vi "2.0.0_BEMF_Calibration.vi"(7 "Data in":T2, 8 "error in (no error)":errorcluster, 9 "AllControls In":T1, 10 "?":T3, 11 "Message Queue out":T4) -> (0 "error out":errorcluster, 1 "Flow":string, 2 "Data":T3, 3 "Message Queue Out":T4, 5 "Data out":T2)   [LabVIEW 2017]
uses:
  DIPC 692 Daemon API/typdef/calibration.ctl
  Depends/AMC/subVIs/TypeDefs/amc_Message Queue.ctl
  Depends/AMC/subVIs/TypeDefs/amc_Message.ctl
  Depends/Tools/Keyed Array/Tools_KeyedArray KeyedArray.ctl
  Ctrls/Data.ctl
  Ctrls/CSV_Data.ctl
  Ctrls/AllControls.ctl
panel:
  in  "Image path":path caption="路径"
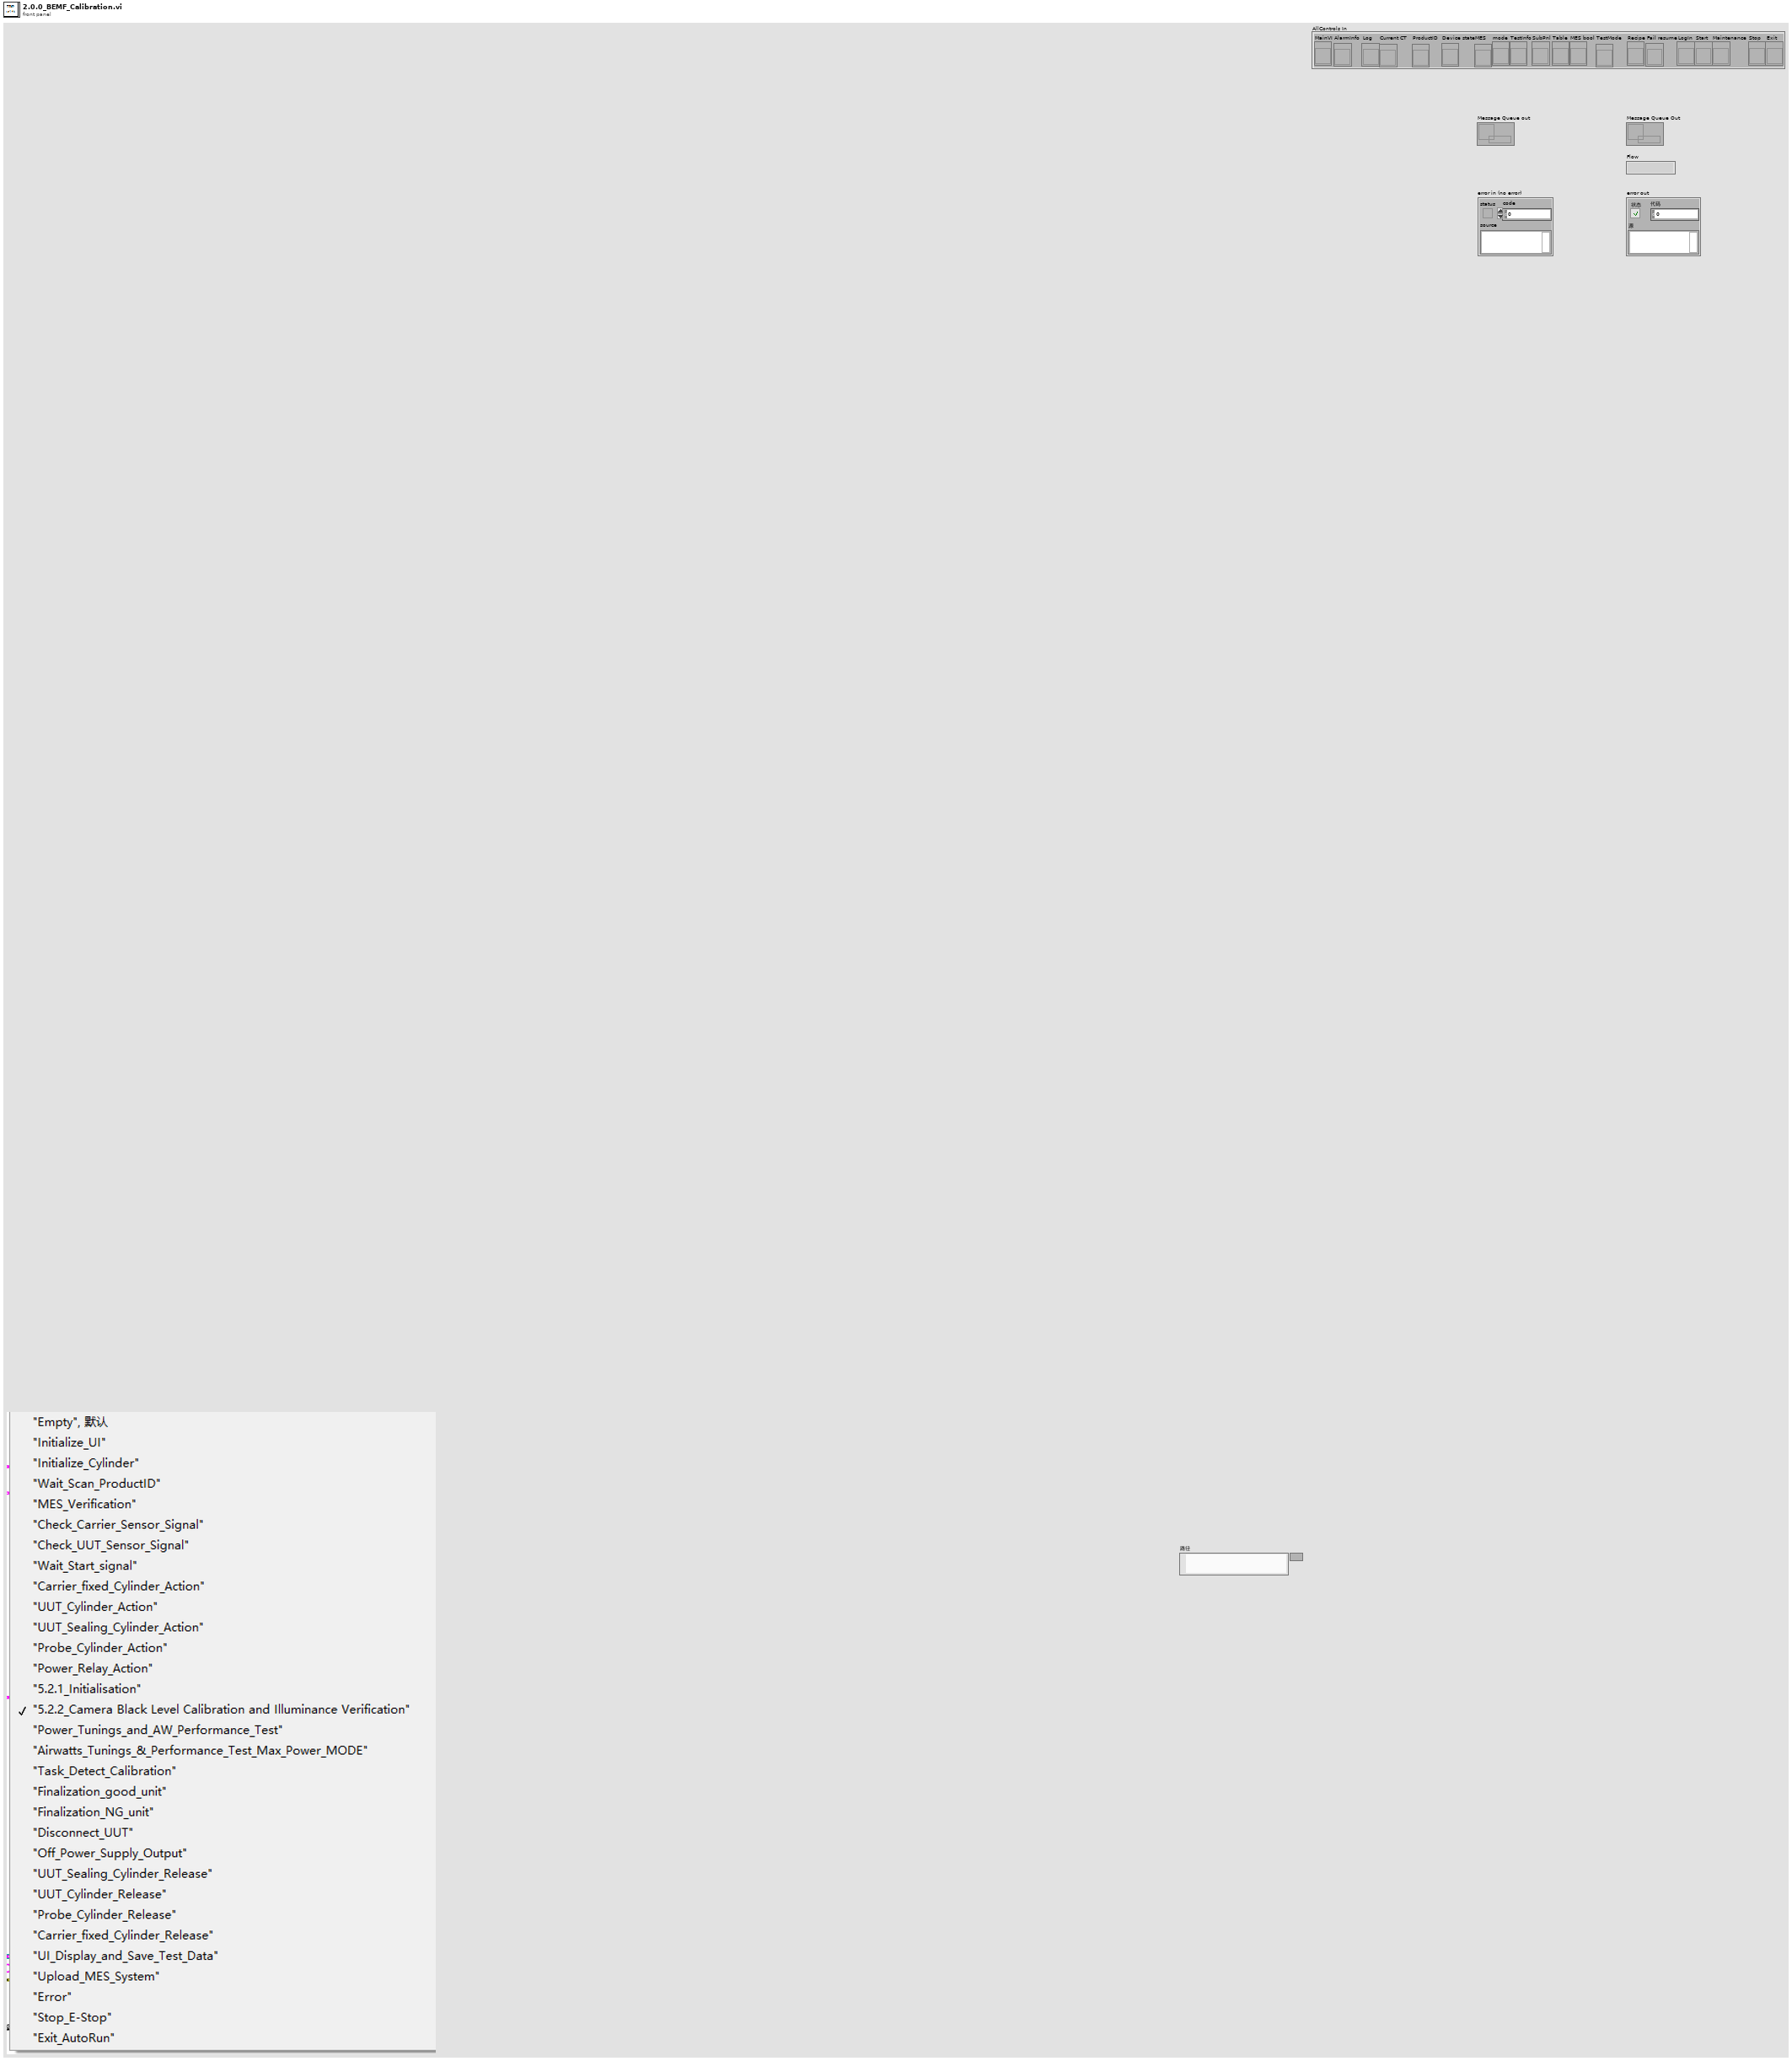
[diagram p1: front panel]
types:
  T1 = typedef "AllControls.ctl" = cluster{"MainVI":refnum<vi>, "AlarmInfo":refnum<vi>, "Log":refnum<vi>, "Current CT":refnum<vi>, "ProductID":refnum<vi>, "Device state":refnum<vi>, "MES":refnum<vi>, "mode":refnum<vi>, "TestInfo":refnum<vi>, "SubPnl":refnum<vi>, "Table":refnum<vi>, "MES bool":refnum<vi>, "TestMode":refnum<vi>, "Recipe":refnum<vi>, "Fail resume":refnum<vi>, "LogIn":refnum<vi>, "Start":refnum<vi>, "Maintenance":refnum<vi>, "Stop":refnum<vi>, "Exit":refnum<vi>}
  T2 = typedef "CSV_Data.ctl" = cluster{"Initialisation":cluster{"LMT - Connect UUT (con COM)":string, "LMT - Software Version (rrel)":string, "LMT - Write SKU file (wskuc)":string, "LMT - SKU file name":string, "Connect UUT DDM":string, "Read DDM EOL Timestamp - Mode":string, "Read DDM EOL Timestamp - Timestamp":string, "Read DDM EOL Timestamp - Rig ID":string, "Read DDM EOL Timestamp - Passmark ID":string, "Read DDM EOL Timestamp - Passmark Rev":string, "Software Version before flashing":string, "Read Hardware Serial":string, "UUT DDM SN":string, "Compare DDM SN with MES SN":string, "Backup PCBA Calibration EEPROM Response - CAL":string, "Flash Firmware Version":string, "Check SW Version":string, "Read DDM SW Version after flashing":string, "Set SKU Config":string, "Ready Status":string, "Set Device Mode to EOL":string, "DDM Parameter - Voltage":string, "DDM Parameter - Current":string, "DDM Parameter - Power":string, "DDM Parameter - Speed":string, "DDM Parameter - Pressure":string, "Tester Parameter - Voltage":string, "Tester Parameter - Current":string, "Tester Parameter - Power":string, "Tester Parameter - Ambient Pressure":string, "Tester Parameter - Ambient Temperature":string, "Calculated Parameter - DDM Pressure Corrected":string, "Calculated Parameter - DDM Real Power":string, "Calculated Parameter - Delta V":string}, "BEMF_Calibration":cluster{"Calibration Result - eol_cold_bemf_temp":string, "DDM Ambient Temp":string, "Restriction Plate Diameter":string, "Calibration Result - eol_bemf_mp_cold_coef_a":string, "Calibration Result - eol_bemf_mp_cold_coef_b":string, "Calibration Result - eol_bemf_mp_cold_coef_c":string, "Calibration Result - eol_bemf_lsi_cold_ref_coeffs":string, "Get - Calibration Result - eol_bemf_lsi_speed":string, "Get - Calibration Result - eol_bemf_lsi_integral_0":string, "Calibration Result - eol_bemf_lsi_integral_1":string, "Get - Calibration Result - eol_bemf_lsi_integral_2":string, "Get - Calibration Result - eol_cold_bemf":string, "Get - Calibration Result - eol_cold_bemf_fisf":string, "Finalise Calibration":string, "Compare -Calibration Result - eol_cold_bemf":string, "Compare -Calibration Result - eol_cold_bemf_fisf":string}, "ECO":cluster{"Reset Power Tune":string, "Reset BEMF FISF Calibration":string, "Restriction Plate Diameter":string, "ECO - Stabilisation Time":string, "ECO - DDM Parameter - Voltage":string, "ECO - DDM Parameter - Current":string, "ECO - DDM Parameter - Power":string, "ECO - DDM Parameter - Measured Power":string, "ECO - DDM Parameter - Speed":string, "ECO - DDM Parameter - Pressure":string, "ECO - Tester Parameter - Voltage":string, "ECO - Tester Parameter - Current":string, "ECO - Tester Parameter - Power":string, "ECO - Tester Parameter - Ambient Pressure":string, "ECO - Tester Parameter - Ambient Temperature":string, "ECO - Tester Parameter - Ambient Humidity":string, "ECO - Calculated Parameter - DDM Pressure Corrected":string, "ECO - Calculated Parameter - DDM Real Power":string, "ECO - Calculated Parameter - Delta V":string, "ECO - Calculated Parameter - Flowrate":string, "ECO - Calculated Parameter - Airwatt":string, "ECO - Formula":string, "PT ECO - Power Tune Mode Status":string}, "BOOST":cluster{"Restriction Plate Diameter":string, "BOOST - Stabilisation Time":string, "BOOST - DDM Parameter - Voltage":string, "BOOST - DDM Parameter - Current":string, "BOOST - DDM Parameter - Power":string, "BOOST - DDM Parameter - Measured Power":string, "BOOST - DDM Parameter - Speed":string, "BOOST - DDM Parameter - Pressure":string, "BOOST - Tester Parameter - Voltage":string, "BOOST - Tester Parameter - Current":string, "BOOST - Tester Parameter - Power":string, "BOOST - Tester Parameter - Ambient Pressure":string, "BOOST - Tester Parameter - Ambient Temperature":string, "BOOST - Tester Parameter - Ambient Humidity":string, "BOOST - Calculated Parameter - DDM Pressure Corrected":string, "BOOST - Calculated Parameter - DDM Real Power":string, "BOOST - Calculated Parameter - Delta V":string, "BOOST - Calculated Parameter - Flowrate":string, "BOOST - Calculated Parameter - Airwatt":string, "BOOST - Get AM Presence":string, "Air Muscle Turn Off Status":string, "BOOST - Air Muscle Calculated Parameter - Airwatt B":string, "BOOST - Air Muscle Calculate Airwatt Delta":string, "PT BOOST - Power Tune Mode Status":string, "Finalise Calibration":string, "ECO - Get AW Calibration value":string, "BOOST - Get AW Calibration value":string}, "MAX":cluster{"Restriction Plate Diameter":string, "MAX - Stabilisation Time":string, "Get Average Delta Tmag (LSIdelta_FISFdelta_LSItmag_FISFtmag_IIRtmag)":string, "Get Average Delta Tmag FISF":string, "MAX - DDM Parameter - Voltage":string, "MAX - DDM Parameter - Current":string, "MAX - DDM Parameter - Power":string, "MAX - DDM Parameter - Measured Power":string, "MAX - DDM Parameter - Speed":string, "MAX - DDM Parameter - Pressure":string, "MAX - Tester Parameter - Voltage":string, "MAX - Tester Parameter - Current":string, "MAX - Tester Parameter - Power":string, "MAX - Tester Parameter - Ambient Pressure":string, "MAX - Tester Parameter - Ambient Temperature":string, "MAX - Tester Parameter - Ambient Humidity":string, "MAX - Calculated Parameter - DDM Pressure Corrected":string, "MAX - Calculated Parameter - DDM Real Power":string, "MAX - Calculated Parameter - Delta V":string, "MAX - Calculated Parameter - Flowrate":string, "MAX - Calculated Parameter - Airwatt":string, "MAX_FISF_Check_Average_Delta_Tmag":string, "MAX - FISF - BEMF Finetune Result":string, "MAX tune - Delta P1":string, "MAX tune - Calculated Parameter - Airwatt":string, "Calculate Delta Airwatts - MAX finetune - Delta P2":string, "MAX finetune - DDM Parameter - Voltage":string, "MAX finetune - DDM Parameter - Current":string, "MAX finetune - DDM Parameter - Power":string, "MAX finetune - DDM Parameter - Measured Power":string, "MAX finetune - DDM Parameter - Speed":string, "MAX finetune - DDM Parameter - Pressure":string, "MAX finetune - Tester Parameter - Voltage":string, "MAX finetune - Tester Parameter - Current":string, "MAX finetune - Tester Parameter - Power":string, "MAX finetune - Tester Parameter - Ambient Pressure":string, "MAX finetune - Tester Parameter - Ambient Temperature":string, "MAX finetune - Tester Parameter - Ambient Humidity":string, "MAX finetune - Calculated Parameter - DDM Pressure Corrected":string, "MAX finetune - Calculated Parameter - DDM Real Power":string, "MAX finetune - Calculated Parameter - Delta V":string, "MAX finetune - Calculated Parameter - Flowrate":string, "MAX finetune - Calculated Parameter - Airwatt":string, "Check Derate Result":string, "Delta Tmag FISF":string, "Get Hot BEMF Result":string, "Calculate delta Pressure":string, "Finalise Calibration":string, "Calculate & Check Delta BEMF":string, "Delta P Airwatts Value":string}, "LL":cluster{"DDM Ambient Temp":string, "Restriction Plate Diameter":string, "LL - DDM Parameter - Voltage":string, "LL - DDM Parameter - Current":string, "LL - DDM Parameter - Power":string, "LL - DDM Parameter - Measured Power":string, "LL - DDM Parameter - Speed":string, "LL - DDM Parameter - Pressure":string, "LL - Tester Parameter - Voltage":string, "LL - Tester Parameter - Current":string, "LL - Tester Parameter - Power":string, "LL - DDM Real Power":string, "LL - Calibrate Task Detect LL":string}, "HL":cluster{"HL - DDM Parameter - Voltage":string, "HL - DDM Parameter - Current":string, "HL - DDM Parameter - Power":string, "HL - DDM Parameter - Measured Power":string, "HL - DDM Parameter - Speed":string, "HL - DDM Parameter - Pressure":string, "HL - Tester Parameter - Voltage":string, "HL - Tester Parameter - Current":string, "HL - Tester Parameter - Power":string, "HL - DDM Real Power":string, "HL - Calibrate Task Detect HL":string}, "LH":cluster{"Restriction Plate Diameter":string, "LH - DDM Parameter - Voltage":string, "LH - DDM Parameter - Current":string, "LH - DDM Parameter - Power":string, "LH - DDM Parameter - Measured Power":string, "LH - DDM Parameter - Speed":string, "LH - DDM Parameter - Pressure":string, "LH - Tester Parameter - Voltage":string, "LH - Tester Parameter - Current":string, "LH - Tester Parameter - Power":string, "LH - DDM Real Power":string, "LH - Calibrate Task Detect LH":string}, "HH":cluster{"HH - DDM Parameter - Voltage":string, "HH - DDM Parameter - Current":string, "HH - DDM Parameter - Power":string, "HH - DDM Parameter - Measured Power":string, "HH - DDM Parameter - Speed":string, "HH - DDM Parameter - Pressure":string, "HH - Tester Parameter - Voltage":string, "HH - Tester Parameter - Current":string, "HH - Tester Parameter - Power":string, "HH - DDM Real Power":string, "HH - Calibrate Task Detect HH":string}, "Inlet Blockage Calibration":cluster{"Inlet Blockage Calibration - DDM Parameter - Voltage":string, "Inlet Blockage Calibration - DDM Parameter - Current":string, "Inlet Blockage Calibration - DDM Parameter - Power":string, "Inlet Blockage Calibration - DDM Parameter - Measured Power":string, "Inlet Blockage Calibration - DDM Parameter - Speed":string, "Inlet Blockage Calibration - DDM Parameter - Pressure":string, "Inlet Blockage Calibration - Tester Parameter - Voltage":string, "Inlet Blockage Calibration - Tester Parameter - Current":string, "Inlet Blockage Calibration - Tester Parameter - Power":string, "Inlet Blockage Calibration - DDM Real Power":string, "Calibration Inlet Blockage_E":string, "Finalise Calibration":string, "Get Task Detect LL":string, "Get Task Detect HL":string, "Get Task Detect LH":string, "Get Task Detect HH":string, "Calibration Inlet Blockage":string, "Calibration eol cold bemf temp":string}, "GOOD":cluster{"GOOD UNIT - Clear EEPROM Error Log":string, "GOOD UNIT - Write Product Timestamp - Mode":string, "GOOD UNIT - Write Product Timestamp - Timestamp":string, "GOOD UNIT - Write Product Timestamp - Rig ID":string, "GOOD UNIT - Write Product Timestamp - Passmark ID":string, "GOOD UNIT - Write Product Timestamp - Passmark Rev":string, "GOOD UNIT - Set Device Mode to PROD":string, "GOOD UNIT - Backup PCBA Calibration EEPROM Response":string, "GOOD UNIT - Check Security Bit":string, "GOOD UNIT - Set Calibration Lock":string, "GOOD UNIT - Get_Calibration_Lock":string, "GOOD UNIT - Disconnect UUT":string}, "NG":cluster{"NG UNIT - Read NVM Error":string, "NG UNIT - Set Device Mode to FCT":string, "NG UNIT - Backup PCBA Calibration EEPROM Response - CAL":string, "NG UNIT - Backup PCBA Calibration EEPROM Response - ERROR":string, "NG UNIT - Backup PCBA Calibration EEPROM Response - USAGE":string, "NG UNIT - Disconnect UUT":string}, "SN":string, "Table":string[][], "Count":cluster{"Total":i32, "OK":i32, "NG":i32, "Yield":dbl}, "Start Time":timestamp, "daemon reference":refnum<k5>, "CT":dbl, "Config":string[][], "OK/NG":bool, "Station ID":string, "MES DDM SN":string, "MES PCBA SN":string, "Retest":string, "Lux":string, "Initialisation_Status":cluster{"LMT - Connect UUT (con COM)":string, "LMT - Software Version (rrel)":string, "LMT - Write SKU file (wskuc)":string, "LMT - SKU file name":string, "Connect UUT DDM":string, "Read DDM EOL Timestamp - Mode":string, "Read DDM EOL Timestamp - Timestamp":string, "Read DDM EOL Timestamp - Rig ID":string, "Read DDM EOL Timestamp - Passmark ID":string, "Read DDM EOL Timestamp - Passmark Rev":string, "Software Version before flashing":string, "Read Hardware Serial":string, "UUT DDM SN":string, "Compare DDM SN with MES SN":string, "Backup PCBA Calibration EEPROM Response - CAL":string, "Flash Firmware Version":string, "Check SW Version":string, "Read DDM SW Version after flashing":string, "Set SKU Config":string, "Ready Status":string, "Set Device Mode to EOL":string, "DDM Parameter - Voltage":string, "DDM Parameter - Current":string, "DDM Parameter - Power":string, "DDM Parameter - Speed":string, "DDM Parameter - Pressure":string, "Tester Parameter - Voltage":string, "Tester Parameter - Current":string, "Tester Parameter - Power":string, "Tester Parameter - Ambient Pressure":string, "Tester Parameter - Ambient Temperature":string, "Calculated Parameter - DDM Pressure Corrected":string, "Calculated Parameter - DDM Real Power":string, "Calculated Parameter - Delta V":string}, "BEMF_Calibration_Status":cluster{"Calibration Result - eol_cold_bemf_temp":string, "DDM Ambient Temp":string, "Restriction Plate Diameter":string, "Calibration Result - eol_bemf_mp_cold_coef_a":string, "Calibration Result - eol_bemf_mp_cold_coef_b":string, "Calibration Result - eol_bemf_mp_cold_coef_c":string, "Calibration Result - eol_bemf_lsi_cold_ref_coeffs":string, "Get - Calibration Result - eol_bemf_lsi_speed":string, "Get - Calibration Result - eol_bemf_lsi_integral_0":string, "Calibration Result - eol_bemf_lsi_integral_1":string, "Get - Calibration Result - eol_bemf_lsi_integral_2":string, "Get - Calibration Result - eol_cold_bemf":string, "Get - Calibration Result - eol_cold_bemf_fisf":string, "Finalise Calibration":string, "Compare -Calibration Result - eol_cold_bemf":string, "Compare -Calibration Result - eol_cold_bemf_fisf":string}, "ECO_Status":cluster{"Reset Power Tune":string, "Reset BEMF FISF Calibration":string, "Restriction Plate Diameter":string, "ECO - Stabilisation Time":string, "ECO - DDM Parameter - Voltage":string, "ECO - DDM Parameter - Current":string, "ECO - DDM Parameter - Power":string, "ECO - DDM Parameter - Measured Power":string, "ECO - DDM Parameter - Speed":string, "ECO - DDM Parameter - Pressure":string, "ECO - Tester Parameter - Voltage":string, "ECO - Tester Parameter - Current":string, "ECO - Tester Parameter - Power":string, "ECO - Tester Parameter - Ambient Pressure":string, "ECO - Tester Parameter - Ambient Temperature":string, "ECO - Tester Parameter - Ambient Humidity":string, "ECO - Calculated Parameter - DDM Pressure Corrected":string, "ECO - Calculated Parameter - DDM Real Power":string, "ECO - Calculated Parameter - Delta V":string, "ECO - Calculated Parameter - Flowrate":string, "ECO - Calculated Parameter - Airwatt":string, "ECO - Formula":string, "PT ECO - Power Tune Mode Status":string}, "BOOST_Status":cluster{"Restriction Plate Diameter":string, "BOOST - Stabilisation Time":string, "BOOST - DDM Parameter - Voltage":string, "BOOST - DDM Parameter - Current":string, "BOOST - DDM Parameter - Power":string, "BOOST - DDM Parameter - Measured Power":string, "BOOST - DDM Parameter - Speed":string, "BOOST - DDM Parameter - Pressure":string, "BOOST - Tester Parameter - Voltage":string, "BOOST - Tester Parameter - Current":string, "BOOST - Tester Parameter - Power":string, "BOOST - Tester Parameter - Ambient Pressure":string, "BOOST - Tester Parameter - Ambient Temperature":string, "BOOST - Tester Parameter - Ambient Humidity":string, "BOOST - Calculated Parameter - DDM Pressure Corrected":string, "BOOST - Calculated Parameter - DDM Real Power":string, "BOOST - Calculated Parameter - Delta V":string, "BOOST - Calculated Parameter - Flowrate":string, "BOOST - Calculated Parameter - Airwatt":string, "BOOST - Get AM Presence":string, "Air Muscle Turn Off Status":string, "BOOST - Air Muscle Calculated Parameter - Airwatt B":string, "BOOST - Air Muscle Calculate Airwatt Delta":string, "PT BOOST - Power Tune Mode Status":string, "Finalise Calibration":string, "ECO - Get AW Calibration value":string, "BOOST - Get AW Calibration value":string}, "MAX_Status":cluster{"Restriction Plate Diameter":string, "MAX - Stabilisation Time":string, "Get Average Delta Tmag (LSIdelta_FISFdelta_LSItmag_FISFtmag_IIRtmag)":string, "Get Average Delta Tmag FISF":string, "MAX - DDM Parameter - Voltage":string, "MAX - DDM Parameter - Current":string, "MAX - DDM Parameter - Power":string, "MAX - DDM Parameter - Measured Power":string, "MAX - DDM Parameter - Speed":string, "MAX - DDM Parameter - Pressure":string, "MAX - Tester Parameter - Voltage":string, "MAX - Tester Parameter - Current":string, "MAX - Tester Parameter - Power":string, "MAX - Tester Parameter - Ambient Pressure":string, "MAX - Tester Parameter - Ambient Temperature":string, "MAX - Tester Parameter - Ambient Humidity":string, "MAX - Calculated Parameter - DDM Pressure Corrected":string, "MAX - Calculated Parameter - DDM Real Power":string, "MAX - Calculated Parameter - Delta V":string, "MAX - Calculated Parameter - Flowrate":string, "MAX - Calculated Parameter - Airwatt":string, "MAX_FISF_Check_Average_Delta_Tmag":string, "MAX - FISF - BEMF Finetune Result":string, "MAX tune - Delta P1":string, "MAX tune - Calculated Parameter - Airwatt":string, "Calculate Delta Airwatts - MAX finetune - Delta P2":string, "MAX finetune - DDM Parameter - Voltage":string, "MAX finetune - DDM Parameter - Current":string, "MAX finetune - DDM Parameter - Power":string, "MAX finetune - DDM Parameter - Measured Power":string, "MAX finetune - DDM Parameter - Speed":string, "MAX finetune - DDM Parameter - Pressure":string, "MAX finetune - Tester Parameter - Voltage":string, "MAX finetune - Tester Parameter - Current":string, "MAX finetune - Tester Parameter - Power":string, "MAX finetune - Tester Parameter - Ambient Pressure":string, "MAX finetune - Tester Parameter - Ambient Temperature":string, "MAX finetune - Tester Parameter - Ambient Humidity":string, "MAX finetune - Calculated Parameter - DDM Pressure Corrected":string, "MAX finetune - Calculated Parameter - DDM Real Power":string, "MAX finetune - Calculated Parameter - Delta V":string, "MAX finetune - Calculated Parameter - Flowrate":string, "MAX finetune - Calculated Parameter - Airwatt":string, "Check Derate Result":string, "Delta Tmag FISF":string, "Get Hot BEMF Result":string, "Calculate delta Pressure":string, "Finalise Calibration":string, "Calculate & Check Delta BEMF":string, "Delta P Airwatts Value":string}, "LL_Status":cluster{"DDM Ambient Temp":string, "Restriction Plate Diameter":string, "LL - DDM Parameter - Voltage":string, "LL - DDM Parameter - Current":string, "LL - DDM Parameter - Power":string, "LL - DDM Parameter - Measured Power":string, "LL - DDM Parameter - Speed":string, "LL - DDM Parameter - Pressure":string, "LL - Tester Parameter - Voltage":string, "LL - Tester Parameter - Current":string, "LL - Tester Parameter - Power":string, "LL - DDM Real Power":string, "LL - Calibrate Task Detect LL":string}, "HL_Status":cluster{"HL - DDM Parameter - Voltage":string, "HL - DDM Parameter - Current":string, "HL - DDM Parameter - Power":string, "HL - DDM Parameter - Measured Power":string, "HL - DDM Parameter - Speed":string, "HL - DDM Parameter - Pressure":string, "HL - Tester Parameter - Voltage":string, "HL - Tester Parameter - Current":string, "HL - Tester Parameter - Power":string, "HL - DDM Real Power":string, "HL - Calibrate Task Detect HL":string}, "LH_Status":cluster{"Restriction Plate Diameter":string, "LH - DDM Parameter - Voltage":string, "LH - DDM Parameter - Current":string, "LH - DDM Parameter - Power":string, "LH - DDM Parameter - Measured Power":string, "LH - DDM Parameter - Speed":string, "LH - DDM Parameter - Pressure":string, "LH - Tester Parameter - Voltage":string, "LH - Tester Parameter - Current":string, "LH - Tester Parameter - Power":string, "LH - DDM Real Power":string, "LH - Calibrate Task Detect LH":string}, "HH_Status":cluster{"HH - DDM Parameter - Voltage":string, "HH - DDM Parameter - Current":string, "HH - DDM Parameter - Power":string, "HH - DDM Parameter - Measured Power":string, "HH - DDM Parameter - Speed":string, "HH - DDM Parameter - Pressure":string, "HH - Tester Parameter - Voltage":string, "HH - Tester Parameter - Current":string, "HH - Tester Parameter - Power":string, "HH - DDM Real Power":string, "HH - Calibrate Task Detect HH":string}, "Inlet Blockage Calibration_Status":cluster{"Inlet Blockage Calibration - DDM Parameter - Voltage":string, "Inlet Blockage Calibration - DDM Parameter - Current":string, "Inlet Blockage Calibration - DDM Parameter - Power":string, "Inlet Blockage Calibration - DDM Parameter - Measured Power":string, "Inlet Blockage Calibration - DDM Parameter - Speed":string, "Inlet Blockage Calibration - DDM Parameter - Pressure":string, "Inlet Blockage Calibration - Tester Parameter - Voltage":string, "Inlet Blockage Calibration - Tester Parameter - Current":string, "Inlet Blockage Calibration - Tester Parameter - Power":string, "Inlet Blockage Calibration - DDM Real Power":string, "Calibration Inlet Blockage_E":string, "Finalise Calibration":string, "Get Task Detect LL":string, "Get Task Detect HL":string, "Get Task Detect LH":string, "Get Task Detect HH":string, "Calibration Inlet Blockage":string, "Calibration eol cold bemf temp":string}, "GOOD_Status":cluster{"GOOD UNIT - Clear EEPROM Error Log":string, "GOOD UNIT - Write Product Timestamp - Mode":string, "GOOD UNIT - Write Product Timestamp - Timestamp":string, "GOOD UNIT - Write Product Timestamp - Rig ID":string, "GOOD UNIT - Write Product Timestamp - Passmark ID":string, "GOOD UNIT - Write Product Timestamp - Passmark Rev":string, "GOOD UNIT - Set Device Mode to PROD":string, "GOOD UNIT - Backup PCBA Calibration EEPROM Response":string, "GOOD UNIT - Check Security Bit":string, "GOOD UNIT - Set Calibration Lock":string, "GOOD UNIT - Get_Calibration_Lock":string, "GOOD UNIT - Disconnect UUT":string}, "NG_Status":cluster{"NG UNIT - Read NVM Error":string, "NG UNIT - Set Device Mode to FCT":string, "NG UNIT - Backup PCBA Calibration EEPROM Response - CAL":string, "NG UNIT - Backup PCBA Calibration EEPROM Response - ERROR":string, "NG UNIT - Backup PCBA Calibration EEPROM Response - USAGE":string, "NG UNIT - Disconnect UUT":string}, "SKU":string, "Plate_Diameter":string, "Alarm":string}
  T3 = typedef "Data.ctl" = cluster{"Initialisation":cluster{"DDM_Parameter":dbl[], "DDM_Parameter_status":bool[], "Get_Tester_Parameter":dbl[], "Get_Tester_Parameter_status":bool[], "Cal_Tester_Parameter":dbl[], "Cal_Tester_Parameter_status":bool[], "sw_version_before_status":bool, "sw_version_after_status":bool, "Set_SKU_Config_With_LMT_status":bool, "FCT_timestamp_status":bool, "LMT_Connect_to_UUT_status":bool}, "BEMF_Calibration":cluster{"Read_ambient_temperature":dbl, "Calibration_Vaule":dbl[], "Calibration_Vaule _B":dbl[], "Calibration_Vaule_status":bool[], "Calibration_Vaule_B_status":bool[]}, "ECO":cluster{"DDM_Parameter":dbl[], "DDM_Parameter_status":bool[], "Get_Tester_Parameter":dbl[], "Get_Tester_Parameter_status":bool[], "Cal_Tester_Parameter":dbl[], "Cal_Tester_Parameter_status":bool[], "DDM_Parameter_after_power_tune":dbl[], "Get_Tester_Parameter_after_power_tune":dbl[], "Cal_Tester_Parameter_after_power_tune":dbl[], "Cal_Tester_Parameter_after_power_tune_status":bool[], "Delta_P":dbl}, "BOOST":cluster{"DDM_Parameter":dbl[], "DDM_Parameter_status":bool[], "Get_Tester_Parameter":dbl[], "Get_Tester_Parameter_status":bool[], "Cal_Tester_Parameter":dbl[], "Cal_Tester_Parameter_status":bool[], "DDM_Parameter_after_power_tune":dbl[], "Get_Tester_Parameter_after_power_tune":dbl[], "Cal_Tester_Parameter_after_power_tune":dbl[], "Cal_Tester_Parameter_after_power_tune_status":bool[], "airwatts_am_off":dbl, "AW_Delta_(AM_on_and_off)":dbl, "AW_Delta_(AM_on_and_off)_Status":bool, "Delta_P":dbl}, "MAX":cluster{"Average_Tmag_Data":cluster{"LSI Delta in degC":dbl, "FISF Delta in degc":dbl, "LSI Tmag in degC":dbl, "Fisf Tmag in degC":dbl, "IIR Tmag in degC":dbl}, "DDM_Parameter":dbl[], "DDM_Parameter_status":bool[], "Get_Tester_Parameter":dbl[], "Get_Tester_Parameter_status":bool[], "Cal_Tester_Parameter":dbl[], "BEMF_Finetune":cluster{"eol_bemf_mp_cold_coef_c":dbl, "eol_cold_bemf_fisf_offset":dbl}, "AW_Tune":cluster{"delta_P1":dbl, "delta_P_Setting":dbl}, "DDM_Parameter_after_Airwatts_Tune":dbl[], "Get_Tester_Parameter_after_Airwatts_Tune":dbl[], "Cal_Tester_Parameter_after_Airwatts_Tune":dbl[], "DDM_Parameter_after_Airwatts_Finetune":dbl[], "Get_Tester_Parameter_after_Airwatts_Finetune":dbl[], "Cal_Tester_Parameter_after_Airwatts_Finetune":dbl[], "AW_Finetune":cluster{"delta_P2":dbl, "delta_P_Setting":dbl}, "Delta_Tmag_after_tune":cluster{"LSI Delta in degC":dbl, "FISF Delta in degc":dbl, "LSI Tmag in degC":dbl, "Fisf Tmag in degC":dbl, "IIR Tmag in degC":dbl}, "Hot Bemf in mV":dbl, "DDM_Pressure":dbl, "Delta_Pressure":dbl, " Cold Bemf in mV":dbl, " delta Bemf":dbl, " delta p":dbl, "Delta_Pressure_status":bool, " delta Bemf_status":bool, "LSI Delta in degC_status":bool, "FISF Delta in degc_status":bool, "Max_check_derate_status_status":bool, "Average_All_data":dbl[][], "Average_Tmag_Data_status":bool[], "Average_Tmag_Data_after_tune_status":bool[], "Cal_Tester_Parameter_status":bool[], "Cal_Tester_Parameter_status_after_Airwatts_Tune":bool[], "Cal_Tester_Parameter_status_after_Airwatts_FineTune":bool[]}, "Task_Detect_Calib":cluster{"LL":cluster{"DDM_Parameter":dbl[], "DDM_Parameter_status":bool[], "Get_Tester_Parameter":dbl[], "Get_Tester_Parameter_status":bool[], "Set_task_detect_A":dbl, "Set_task_detect_A_Status":bool}, "HL":cluster{"DDM_Parameter":dbl[], "DDM_Parameter_status":bool[], "Get_Tester_Parameter":dbl[], "Get_Tester_Parameter_status":bool[], "Set_task_detect_B":dbl, "Set_task_detect_B_Status":bool}, "LH":cluster{"DDM_Parameter":dbl[], "DDM_Parameter_status":bool[], "Get_Tester_Parameter":dbl[], "Get_Tester_Parameter_status":bool[], "Set_task_detect_C":dbl, "Set_task_detect_C_Status":bool}, "HH":cluster{"DDM_Parameter":dbl[], "DDM_Parameter_status":bool[], "Get_Tester_Parameter":dbl[], "Get_Tester_Parameter_status":bool[], "Set_task_detect_D":dbl, "Read_and_check_calibration_Status":bool[], "Set_task_detect_D_Status":bool}, "Get_eol_inlet_blockage_E":dbl, "Calib_vaule":cluster{"Get_task_detect_LL":dbl, "Get_task_detect_HL":dbl, "Get_task_detect_LH":dbl, "Get_task_detect_HH":dbl, "eol_inlet_blockage":dbl, "eol_code_bemf_temp":dbl}, "calibrated temp":dbl, "Inlet_Blockage_Calibration":cluster{"DDM_Parameter":dbl[], "DDM_Parameter_status":bool[], "Get_Tester_Parameter":dbl[], "Get_Tester_Parameter_status":bool[]}, "Get_eol_inlet_blockage_E_Status":bool}, "good":cluster{"Write_Product_TS":cluster{"TIMESTAMP":i64, "RIG_ID":i64, "PASSMARK_ID":i64, "PASSMARK_REV":i64}, "Read_Product_TS":cluster{"TIMESTAMP":i64, "RIG_ID":i64, "PASSMARK_ID":i64, "PASSMARK_REV":i64}, "Good_Check_Secuity_Bit_Stauts":bool}}
  T4 = typedef "amc_Message Queue.ctl" = refnum<queue>
  T5 = typedef "HD Config.ctl" = cluster{" PC":cluster{"PC Address":u8[], "PC Port":i32}, "FCO":cluster{"COM":refnum<visa-resource-name>, "Baudrate":u32}, "DC Power ":cluster{"COM":refnum<visa-resource-name>, "Baudrate":u32}, "PW3336":cluster{"COM":refnum<visa-resource-name>, "Baudrate":u32}, "Lefoo":cluster{"COM":refnum<visa-resource-name>, "Baudrate":u32}, "Tempt&Hum":cluster{"COM":refnum<visa-resource-name>, "Baudrate":u32}, "DIPC":cluster{"COM":refnum<visa-resource-name>}, "Daemon":cluster{"IP Address":string, "Port":u16, "Retry":u16}, "Motor":cluster{"COM":refnum<visa-resource-name>, "Baudrate":u32}, "Fail_resume_mode":bool, "GRR":bool}
  T6 = cluster{"getVersion":string, "Start Test mode":string, "Start camera test mode P1":string, "get one RAW Image":string, "Start camera test mode P0":string, "Stop Test Mode":string, "Stop Camera":string}
  T7 = typedef "calibration.ctl" = string
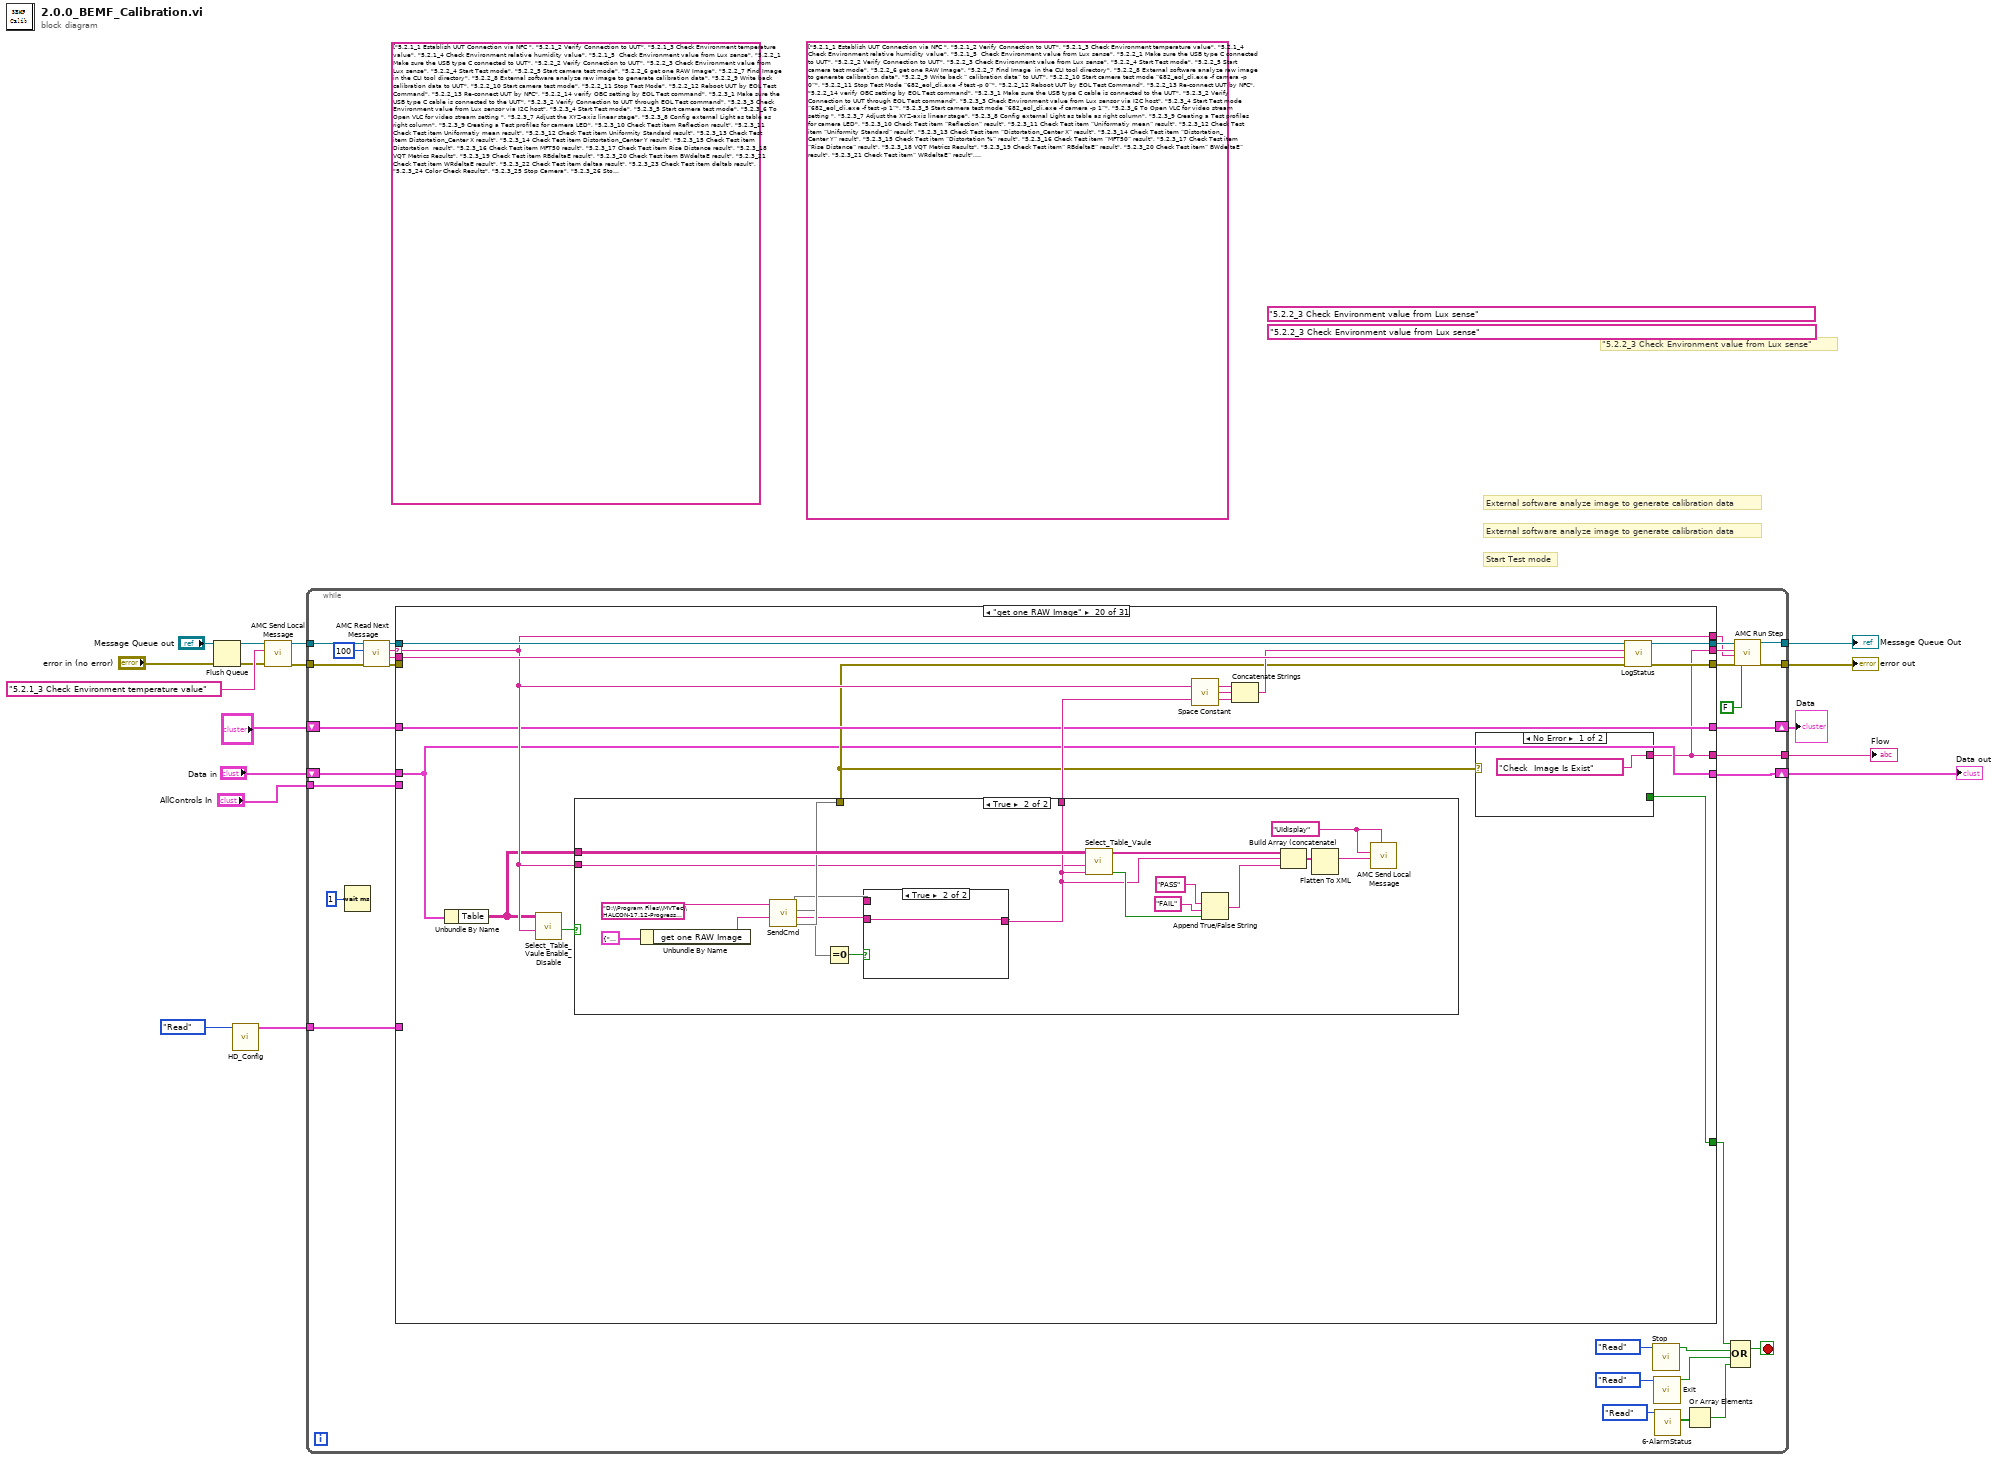
[diagram p0: block diagram]
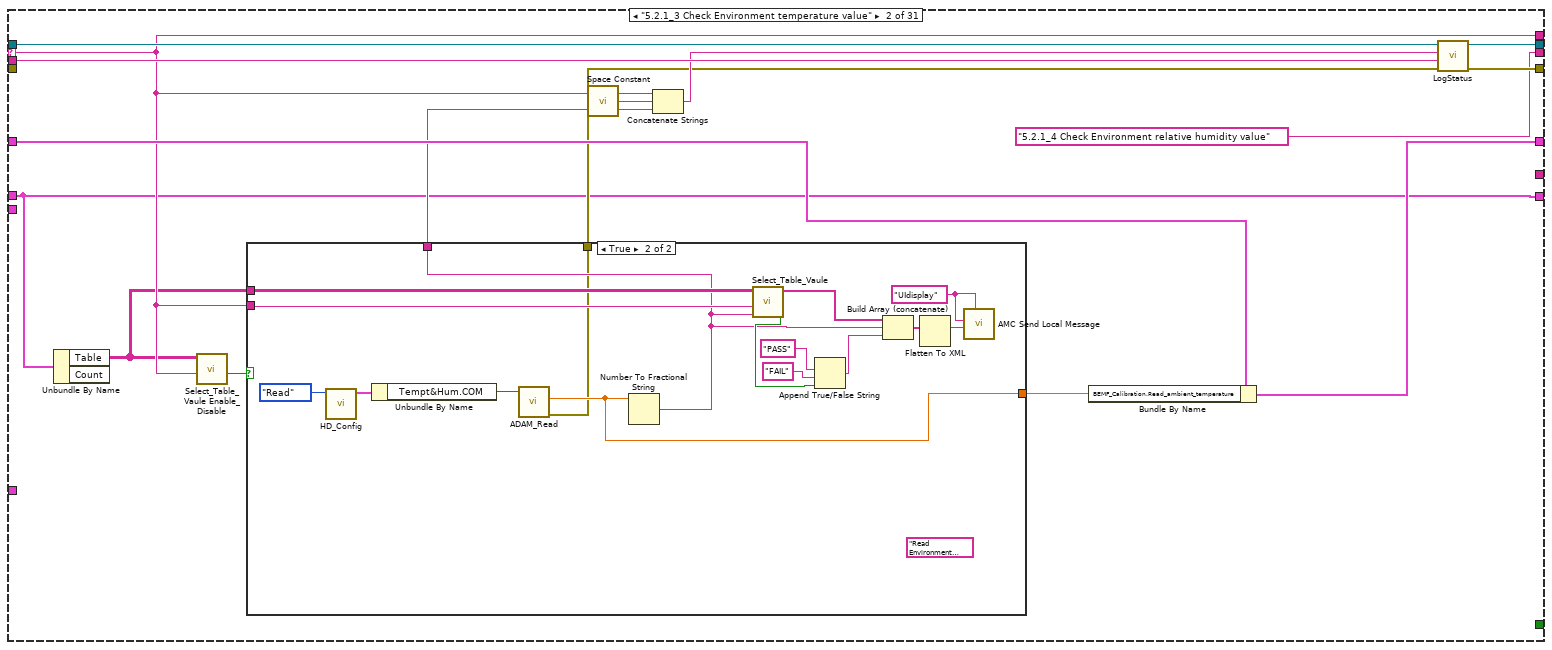
[diagram p3: hidden frame]
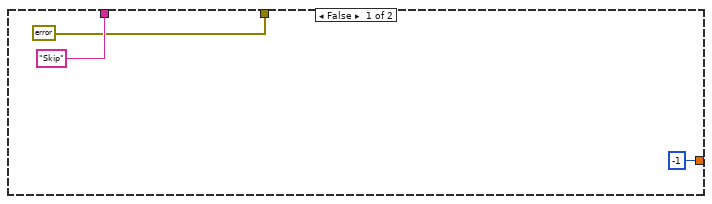
[diagram p4: hidden frame]
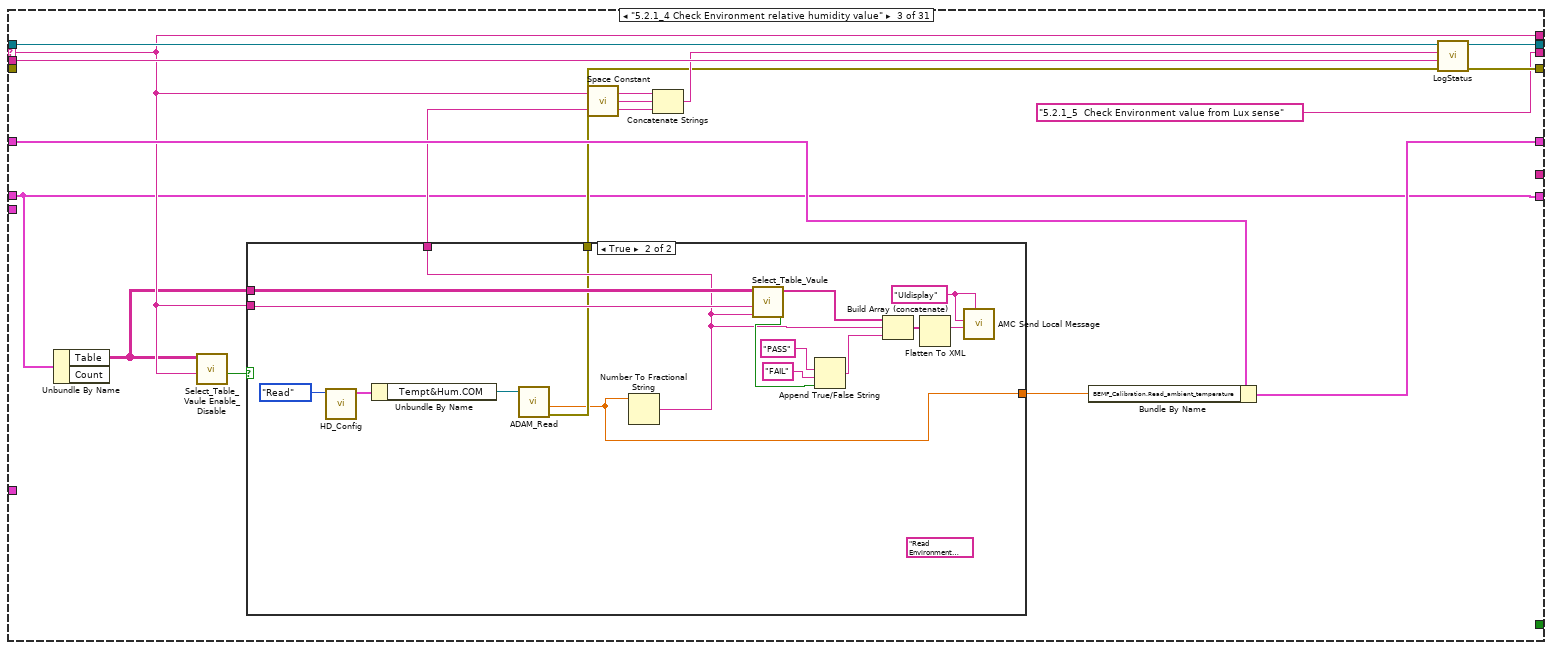
[diagram p5: hidden frame]
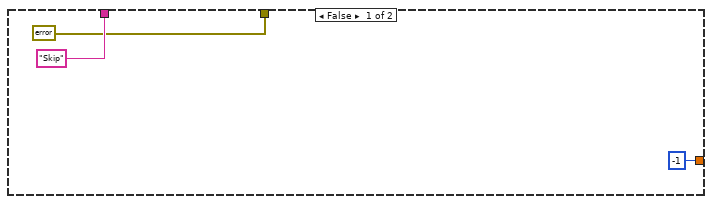
[diagram p6: hidden frame]
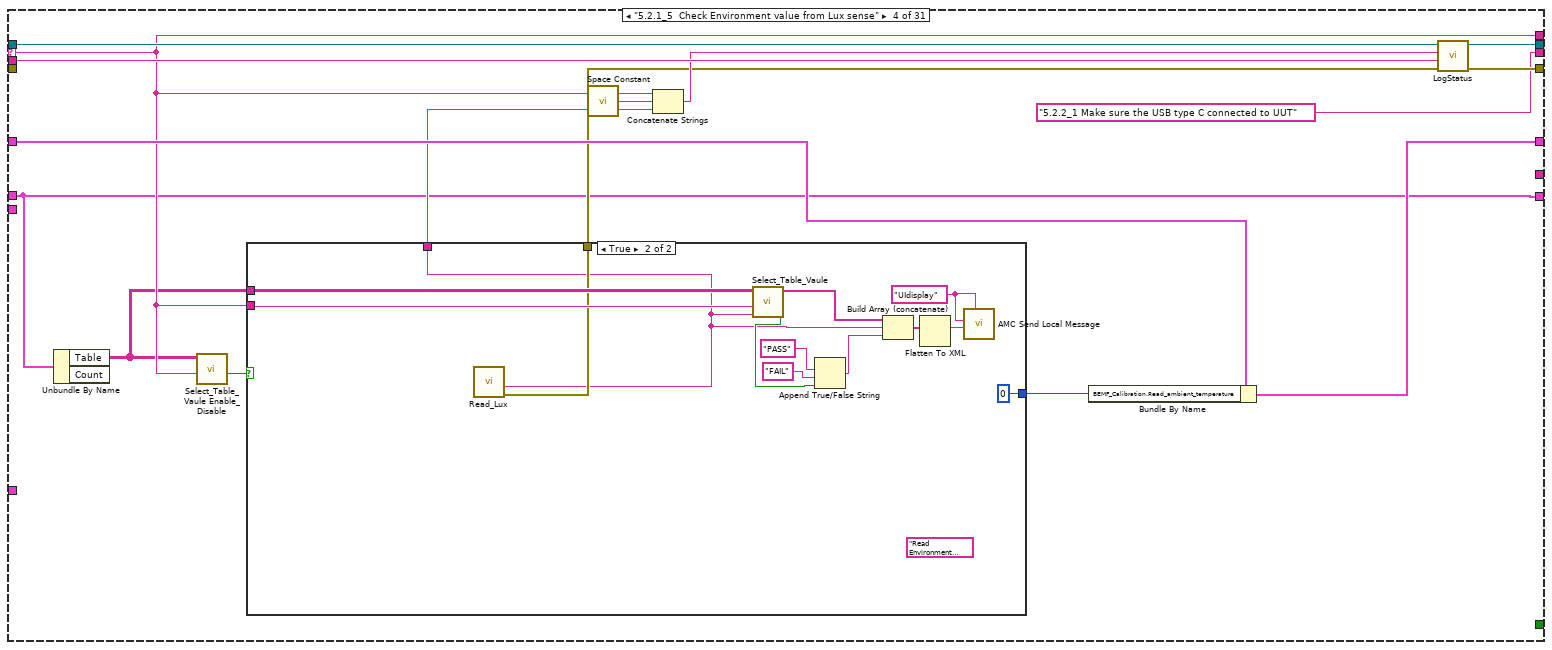
[diagram p7: hidden frame]
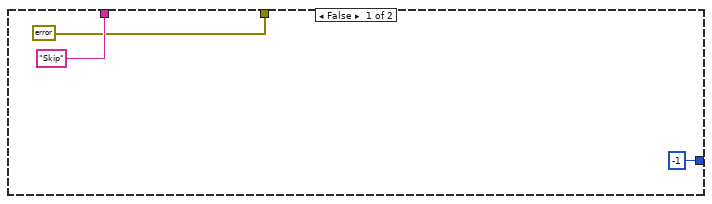
[diagram p8: hidden frame]
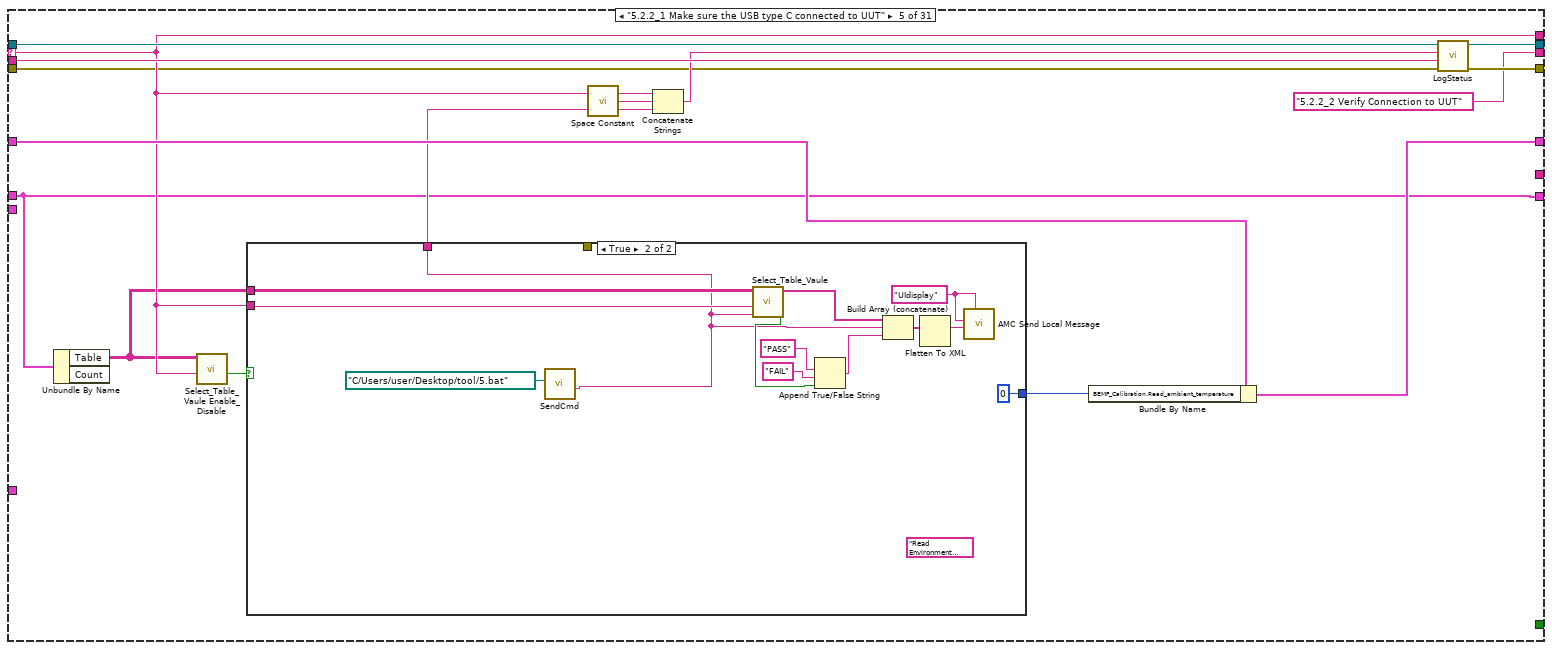
[diagram p9: hidden frame]
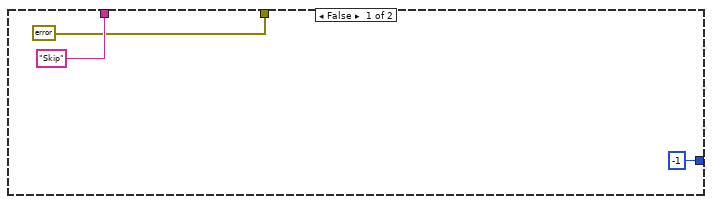
[diagram p10: hidden frame]
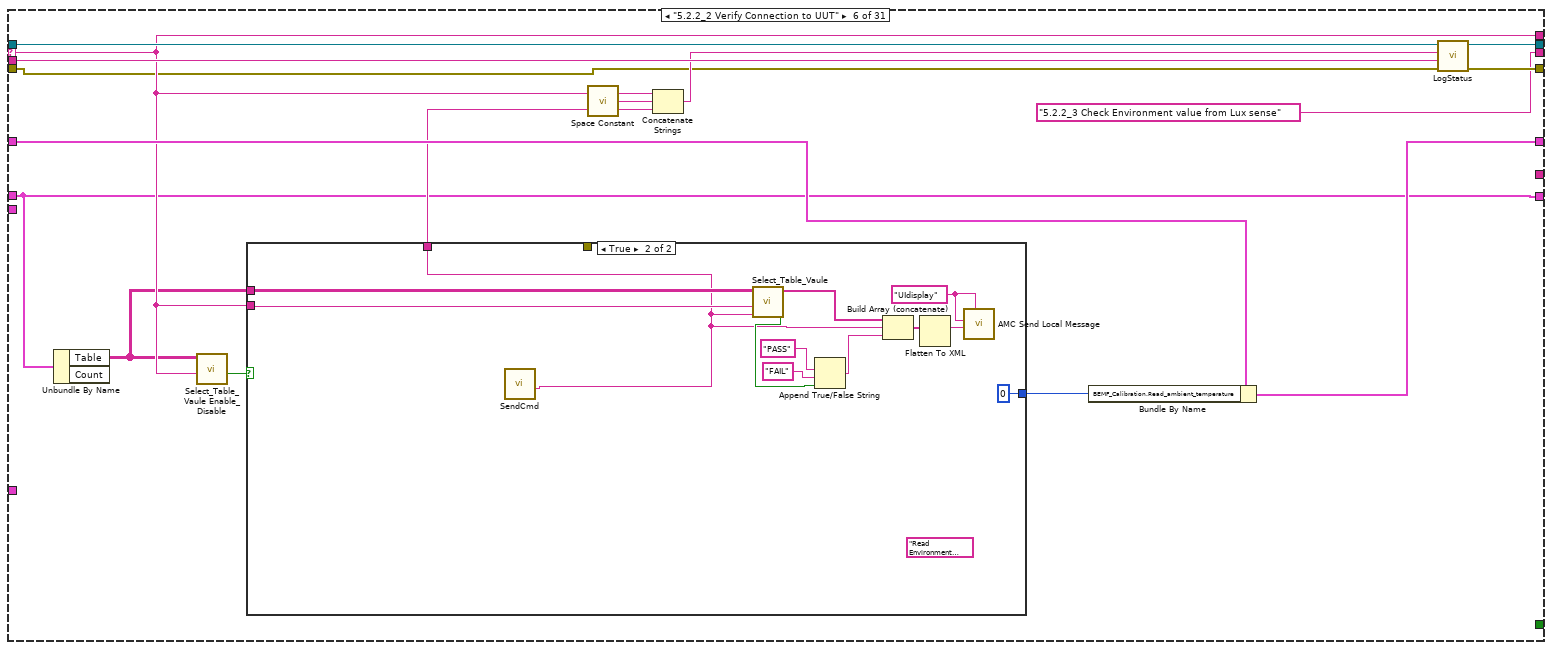
[diagram p11: hidden frame]
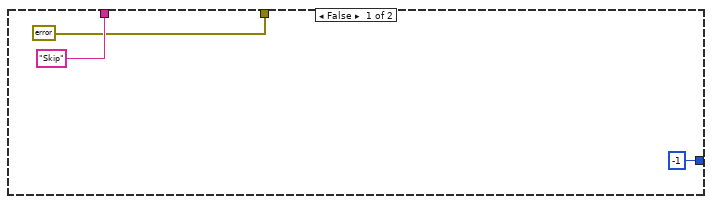
[diagram p12: hidden frame]
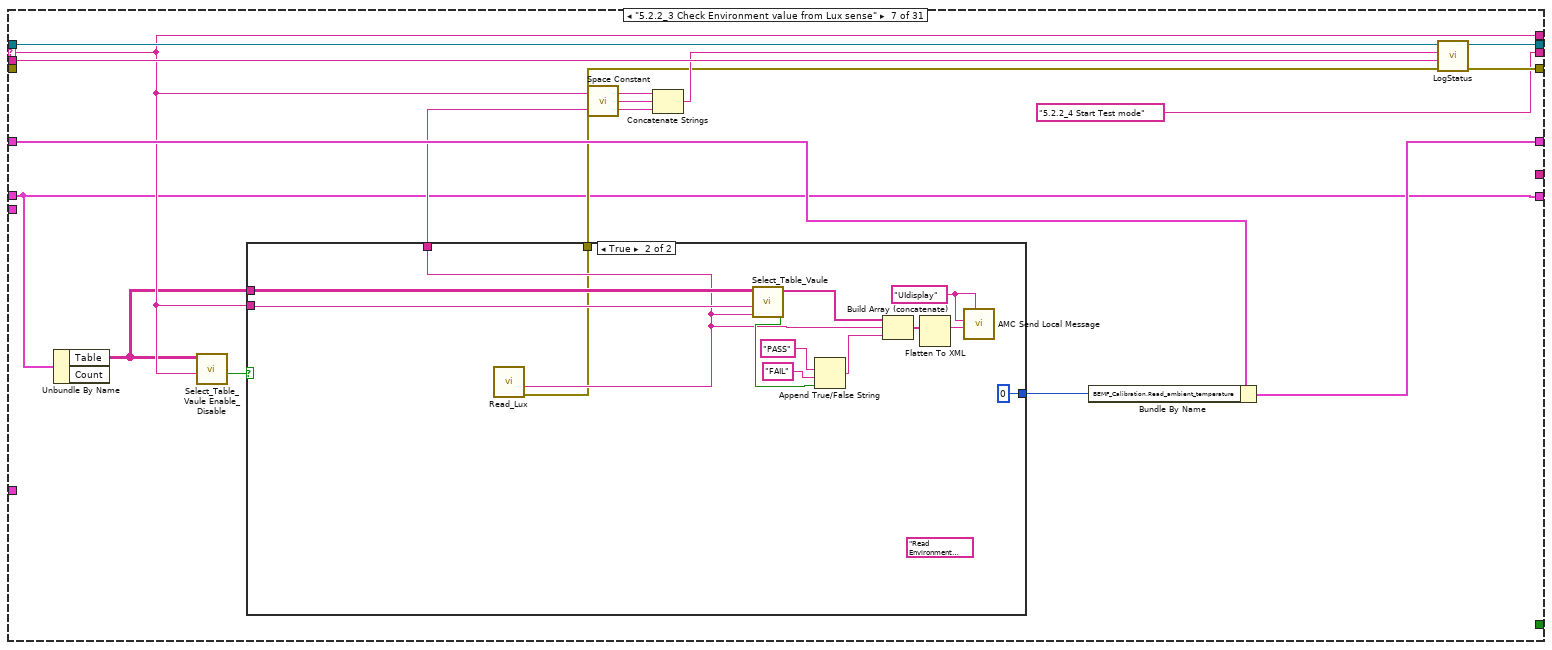
[diagram p13: hidden frame]
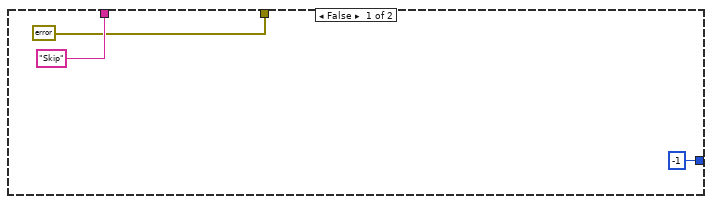
[diagram p14: hidden frame]
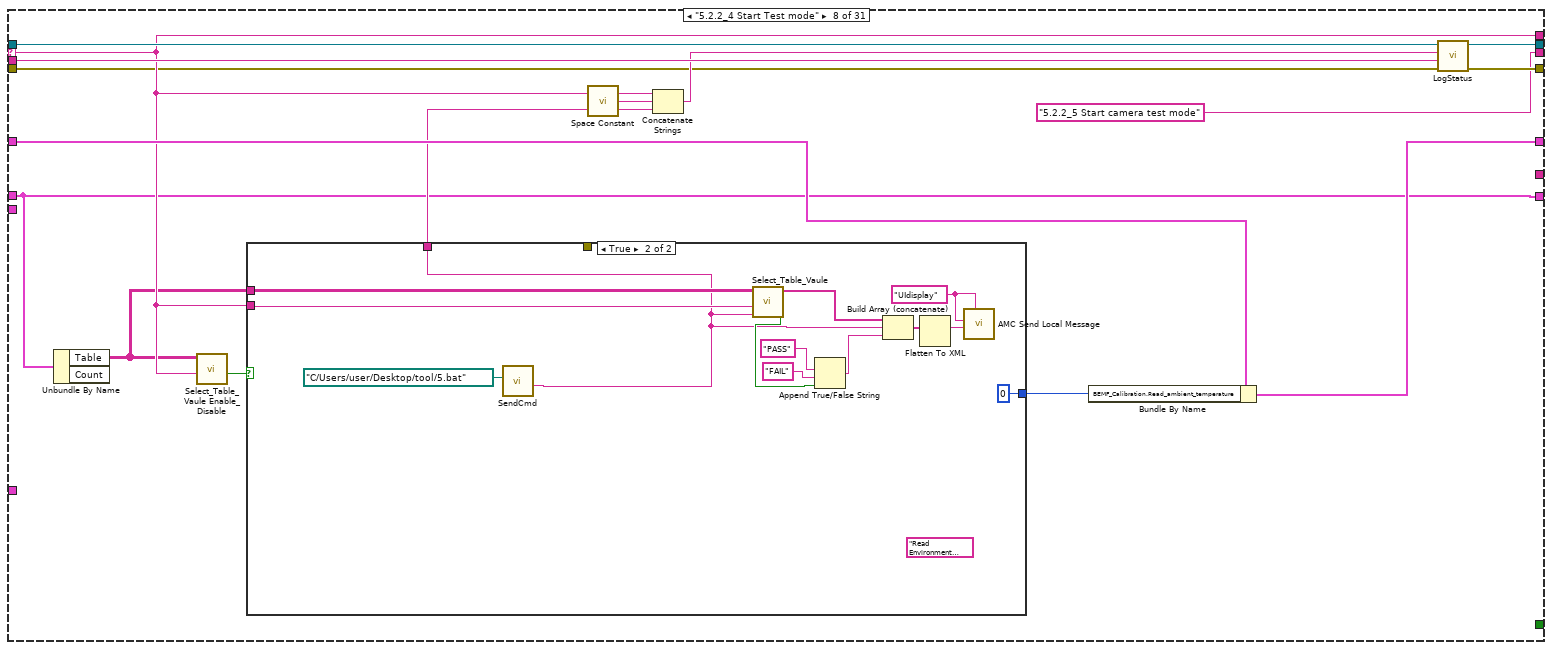
[diagram p15: hidden frame]
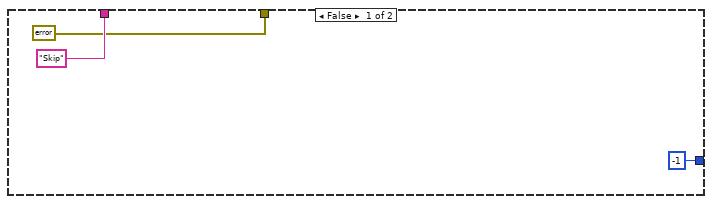
[diagram p16: hidden frame]
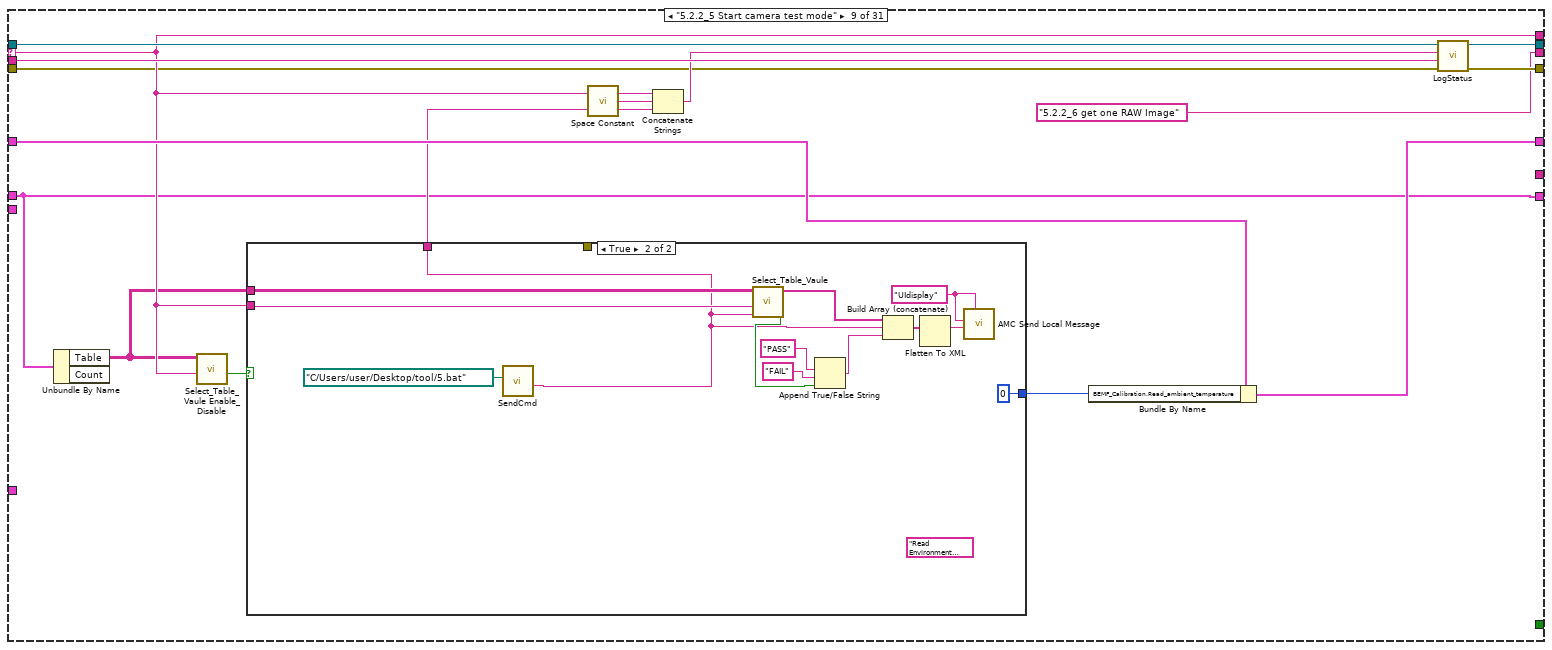
[diagram p17: hidden frame]
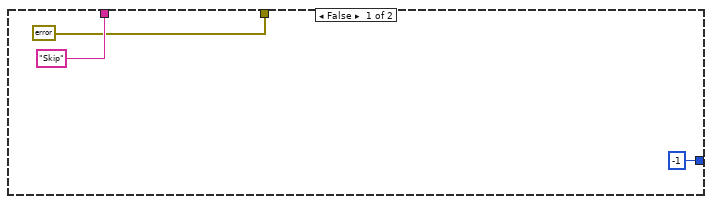
[diagram p18: hidden frame]
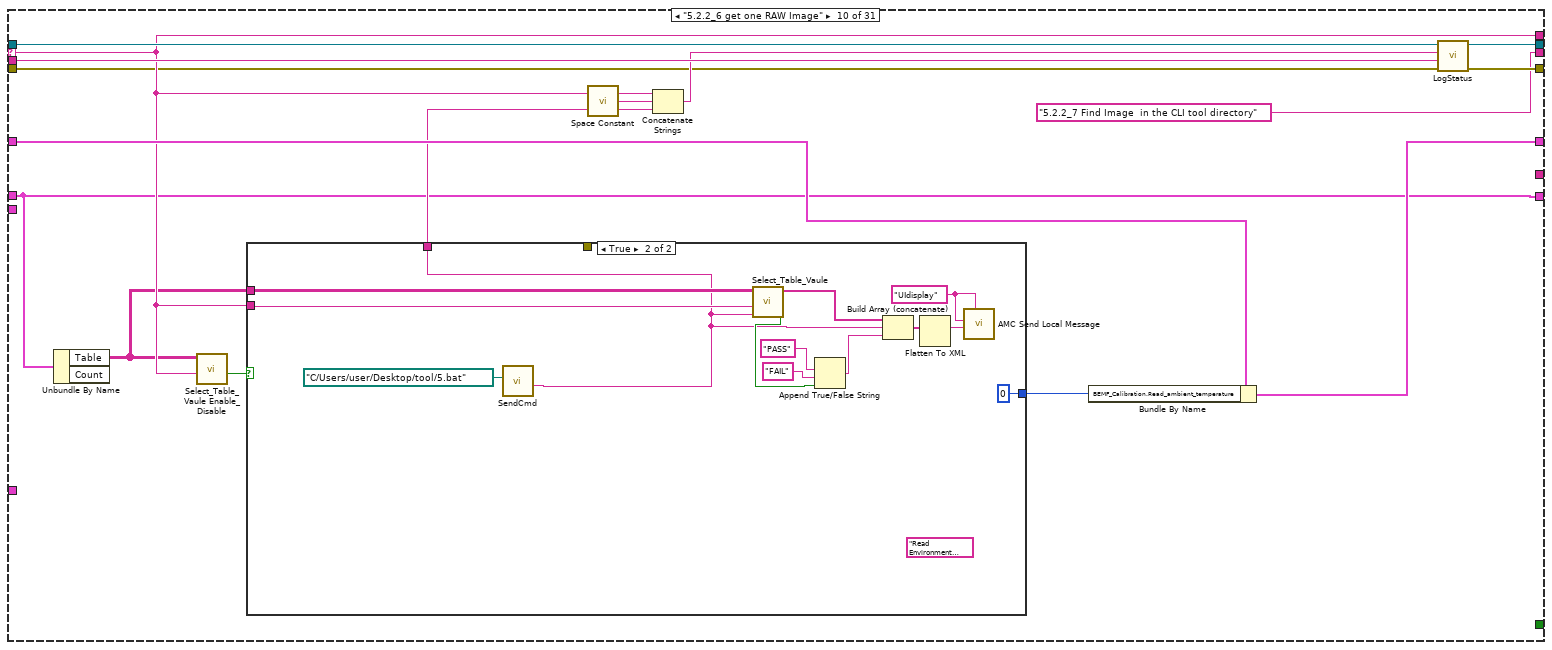
[diagram p19: hidden frame]
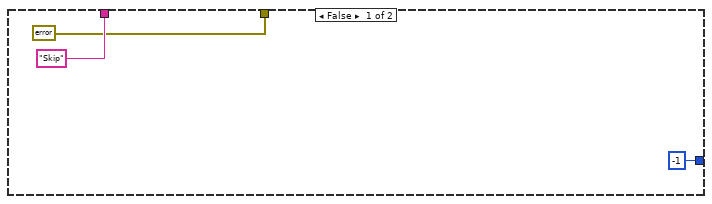
[diagram p20: hidden frame]
diagram:
  (unwired) "5.2.2_3 Check Environment value from Lux sense"
  (unwired) "5.2.2_3 Check Environment value from Lux sense"
  (unwired) string[] ["5.2.1_1 Establish UUT Connection via NFC ", "5.2.1_2 Verify Connection to UUT", "5.2.1_3 Check Environment temperature value", "5.2.1_4 Check Environment relative humidity value", "5.2.1_5  Check Environment value from Lux sense", "5.2.2_1 Make sure the USB type C connected to UUT", "5.2.2_2 Verify Connection to UUT", "5.2.2_3 Check Environment value from Lux sense", "5.2.2_4 Start Test mode", "5.2.2_5 Start camera test mode", "5.2.2_6 get one RAW Image", "5.2.2_7 Find Image  in the CLI tool directory", "5.2.2_8 External software analyze raw image to generate calibration data", "5.2.2_9 Write back calibration data to UUT", "5.2.2_10 Start camera test mode", "5.2.2_11 Stop Test Mode", "5.2.2_12 Reboot UUT by EOL Test Command", "5.2.2_13 Re-connect UUT by NFC", "5.2.2_14 verify OBC setting by EOL Test command", "5.2.3_1 Make sure the USB type C cable is connected to the UUT", "5.2.3_2 Verify Connection to UUT through EOL Test command", "5.2.3_3 Check Environment value from Lux sensor via I2C host", "5.2.3_4 Start Test mode", "5.2.3_5 Start camera test mode", "5.2.3_6 To Open VLC for video stream setting ", "5.2.3_7 Adjust the XYZ-axis linear stage", "5.2.3_8 Config external Light as table as right column", "5.2.3_9 Creating a Test profiles for camera LED", "5.2.3_10 Check Test item Reflection result", "5.2.3_11 Check Test item Uniformatiy mean result", "5.2.3_12 Check Test item Uniformity Standard result", "5.2.3_13 Check Test item Distortation_Center X result", "5.2.3_14 Check Test item Distortation_Center Y result", "5.2.3_15 Check Test item Distortation  result", "5.2.3_16 Check Test item MFT50 result", "5.2.3_17 Check Test item Rise Distance result", "5.2.3_18 VQT Metrics Results", "5.2.3_19 Check Test item RBdeltaE result", "5.2.3_20 Check Test item BWdeltaE result", "5.2.3_21 Check Test item WRdeltaE result", "5.2.3_22 Check Test item deltaa result", "5.2.3_23 Check Test item deltab result", "5.2.3_24 Color Check Results", "5.2.3_25 Stop Camera", "5.2.3_26 Stop Test mode", "5.2.3_27 Shutdown UUT"] ("subarray")
  (unwired) string[] ["5.2.1_1 Establish UUT Connection via NFC ", "5.2.1_2 Verify Connection to UUT", "5.2.1_3 Check Environment temperature value", "5.2.1_4 Check Environment relative humidity value", "5.2.1_5  Check Environment value from Lux sense", "5.2.2_1 Make sure the USB type C connected to UUT", "5.2.2_2 Verify Connection to UUT", "5.2.2_3 Check Environment value from Lux sense", "5.2.2_4 Start Test mode", "5.2.2_5 Start camera test mode", "5.2.2_6 get one RAW Image", "5.2.2_7 Find Image  in the CLI tool directory", "5.2.2_8 External software analyze raw image to generate calibration data", "5.2.2_9 Write back “ calibration data” to UUT", "5.2.2_10 Start camera test mode “682_eol_cli.exe -f camera -p 0”", "5.2.2_11 Stop Test Mode “682_eol_cli.exe -f test -p 0”", "5.2.2_12 Reboot UUT by EOL Test Command", "5.2.2_13 Re-connect UUT by NFC", "5.2.2_14 verify OBC setting by EOL Test command", "5.2.3_1 Make sure the USB type C cable is connected to the UUT", "5.2.3_2 Verify Connection to UUT through EOL Test command", "5.2.3_3 Check Environment value from Lux sensor via I2C host", "5.2.3_4 Start Test mode “682_eol_cli.exe -f test -p 1”", "5.2.3_5 Start camera test mode “682_eol_cli.exe -f camera -p 1”", "5.2.3_6 To Open VLC for video stream setting ", "5.2.3_7 Adjust the XYZ-axis linear stage", "5.2.3_8 Config external Light as table as right column", "5.2.3_9 Creating a Test profiles for camera LED", "5.2.3_10 Check Test item “Reflection” result", "5.2.3_11 Check Test item “Uniformatiy mean” result", "5.2.3_12 Check Test item “Uniformity Standard” result", "5.2.3_13 Check Test item “Distortation_Center X” result", "5.2.3_14 Check Test item “Distortation_Center Y” result", "5.2.3_15 Check Test item “Distortation %” result", "5.2.3_16 Check Test item “MFT50” result", "5.2.3_17 Check Test item “Rise Distance” result", "5.2.3_18 VQT Metrics Results", "5.2.3_19 Check Test item” RBdeltaE” result", "5.2.3_20 Check Test item” BWdeltaE” result", "5.2.3_21 Check Test item” WRdeltaE” result", "5.2.3_22 Check Test item” deltaa” result", "5.2.3_23 Check Test item” deltab” result ", "5.2.3_24 Color Check Results", "5.2.3_25 Stop Camera “682_eol_cli.exe -f camera -p 0”", "5.2.3_26 Stop Test mode “682_eol_cli.exe -f test -p 0”", "5.2.3_27 Shutdown UUT"] ("subarray")
  # "\"5.2.2_3 Check Environment value from Lux sense\""
  # "External software analyze image to generate calibration data"
  # "External software analyze image to generate calibration data"
  # "Start Test mode"
  n1 = Flush Queue(queue="Message Queue out") -> (queue out=w6:T4)  [unwired: 1 in, 2 out]
  n2 = call "HD_Config.vi"("Step"=enum16{"Initial", "Write", "Read"}."Read") -> ("HD Config out"=w8:T5)  [unwired: 9 in, 1 out]
  n3 = call "AMC Send Local Message.vi"("error in (no error)"="error in (no error)", "Message Name"="5.2.1_3 Check Environment temperature value", "Message Queue in"=w6) -> ("error out"=w13:errorcluster, "Message Queue out"=w14:T4)  [unwired: 7 in]
  n4 = while {
    tunnel: w14 -> [w47]
    tunnel: [w43] -> w5
    tunnel: w13 -> [w41]
    tunnel: [w38] -> w4
    shift-right: [w34] -> w10
    shift-left: "?" -> [w35]
    tunnel: w8 -> [w33]
    tunnel: [w29] -> w7
    shift-right: [w21] -> w2
    shift-left: "Data in" -> [w22]
    tunnel: "AllControls In" -> [w20]
    stop <- w23 stop-if-true
    n5 = Wait (ms)(milliseconds to wait=u32 1 ("等待时间（毫秒）")) -> ()  [unwired: 1 out]
    n6 = call "AMC Read Next Message.vi"("error in (no error)"=w41, "timeout (1ms)"=100, "Message Queue in"=w47) -> ("error out"=w40:errorcluster, "Message Value"=w31:string, "Message Name"=w45:string, "Message Queue out"=w46:T4)  [unwired: 1 in, 4 out]
    n7 = case shown="\"get one RAW Image\"" w45 {
      selector: w45 -> [_ w57 w91 w125 w156 w187 w217 w248 w279 w310 w341 w372 w402 w432 w462 w492 w522 w553 w585 w615 w654 w688 w723 w758 w797 w836 w875 w914 w997 w1085 w1151]
      tunnel: w46 -> [w51 w66 w100 w134 w165 w196 w226 w257 w288 w319 w350 w381 w411 w441 w471 w501 w531 w562 w591 w621 w660 w694 w729 w764 w803 w842 w881 w920 w1006 w1092 w1159]
      tunnel: [w51 w66 w100 w134 w165 w196 w226 w257 w288 w319 w350 w381 w411 w441 w471 w501 w531 w562 w591 w621 w660 w694 w729 w764 w803 w842 w881 w920 w1006 w1092 w1159] -> w44
      tunnel: w40 -> [w50 _ _ _ w151 w182 _ w243 w274 w305 w336 w367 w397 w427 w457 w487 w517 w547 w578 _ _ _ _ _ _ _ _ _ _ _ _]
      tunnel: [w50 w65 w99 w133 w164 w195 w225 w256 w287 w318 w349 w380 w410 w440 w470 w500 w530 w561 w590 w620 w659 w693 w728 w763 w802 w841 w880 w919 w1005 w1091 w1158] -> w39
      tunnel: [_ _ _ _ _ _ _ _ _ _ _ _ _ _ _ _ _ TRUE w584 w614 w653 w687 w722 w757 w796 w835 w874 w913 w987 w1080 TRUE] -> w24
      tunnel: w35 -> [w49 w63 w97 w131 w162 w193 w223 w254 w285 w316 w347 w378 w408 w438 w468 w498 w528 w559 w581 w611 w650 w684 w719 w754 w793 w832 w871 w910 w1002 w1078 w1156]
      tunnel: [w49 w62 w96 w130 w161 w192 w222 w253 w284 w315 w346 w377 w407 w437 w467 w497 w527 w558 w581 w611 w650 w684 w719 w754 w793 w832 w871 w910 w1001 w1078 w1155] -> w34
      tunnel: w31 -> [_ w64 w98 w132 w163 w194 w224 w255 w286 w317 w348 w379 w409 w439 w469 w499 w529 w560 w589 w619 w658 w692 w727 w762 w801 w840 w879 w918 w1004 w1090 w1157]
      tunnel: [_ w57 w91 w125 w156 w187 w217 w248 w279 w310 w341 w372 w402 w432 w462 w492 w522 w553 w585 w615 w654 w688 w723 w758 w797 w836 w875 w914 w997 w1085 w1151] -> w30
      tunnel: w33 -> [_ _ _ _ _ _ _ _ _ _ _ _ _ _ _ _ _ _ _ _ _ _ _ _ _ _ _ _ _ _ _]
      tunnel: [_ "5.2.1_4 Check Environment relative humidity value" "5.2.1_5  Check Environment value from Lux sense" "5.2.2_1 Make sure the USB type C connected to UUT" "5.2.2_2 Verify Connection to UUT" "5.2.2_3 Check Environment value from Lux sense" "5.2.2_4 Start Test mode" "5.2.2_5 Start camera test mode" "5.2.2_6 get one RAW Image" "5.2.2_7 Find Image  in the CLI tool directory" "5.2.2_8 External software analyze raw image to generate calibration data" "5.2.2_9 Write back calibration data to UUT" "5.2.2_10 Start camera test mode" "5.2.2_11 Stop Test Mode" "5.2.2_12 Reboot UUT by EOL Test Command" "5.2.2_13 Re-connect UUT by NFC" "5.2.2_14 verify OBC setting by EOL Test command" "5.2.3_Camera Vision Quality Test" w579 w608 w647 w681 w716 w751 w790 w829 w868 w907 w993 "Calibration_Read_and_check_Calibration_value_B" w1149] -> w32
      tunnel: [_ _ _ _ _ _ _ _ _ _ _ _ _ _ _ _ _ _ w579 w608 w647 w681 w716 w751 w790 w829 w868 w907 w993 w1081 w1149] -> w29
      tunnel: w22 -> [w48 w52 w86 w120 w153 w183 w212 w244 w275 w306 w337 w368 w398 w428 w458 w488 w518 w549 w580 w609 w648 w682 w717 w752 w791 w830 w869 w908 w986 w1077 w1131]
      tunnel: [w48 w52 w86 w120 w153 w183 w212 w244 w275 w306 w337 w368 w398 w428 w458 w488 w518 w549 w580 w609 w648 w682 w717 w752 w791 w830 w869 w908 w982 w1074 w1130] -> w21
      tunnel: w20 -> [_ _ _ _ _ _ _ _ _ _ _ _ _ _ _ _ _ _ _ _ _ _ _ _ _ _ _ _ w974 w1065 w1132]
      frame "假", Default {
      }
      frame "5.2.1_3 Check Environment temperature value" {
        n8 = Unbundle By Name(w52) -> ("Table"=w56:string[][])  [unwired: 1 out]
        n9 = call "Select_Table_Vaule Enable_Disable.vi"("Action"=w57, "Table"=w56) -> ("Enable"=w58:bool)  [unwired: 8 in, 1 out]
        n10 = case shown="True" w58 {
          tunnel: ["Skip" ("response") w72] -> w59
          tunnel: w57 -> [_ w80]
          tunnel: w56 -> [_ w79]
          tunnel: [errorcluster {"status"=FALSE, "code"=0, "source"=""} ("错误输出") w70] -> w53
          tunnel: [-1 w71] -> w54
          frame False {
          }
          frame True {
            (unwired) "Read Environment Illuminance Value Success"
            w85 = "UIdisplay" ("Process (\"\" - local)")
            n11 = call "HD_Config.vi"("Step"=enum16{"Initial", "Write", "Read"}."Read") -> ("HD Config out"=w75:T5)  [unwired: 9 in, 1 out]
            n12 = Unbundle By Name(w75) -> ("Tempt&Hum.COM"=w73:refnum<visa-resource-name>)
            n13 = call "ADAM_Read.vi"("VISA resource name"=w73) -> ("error out"=w70:errorcluster, "temperature"=w71:dbl)  [unwired: 7 in, 2 out]
            n14 = Number To Fractional String(number=w71) -> (F-format string=w72:string)  [unwired: 3 in]
            n15 = call "Select_Table_Vaule.vi"("Vaule"=w72, "Action"=w80, "Table"=w79) -> ("Result"=w76:bool, "vaule"=w78:string[])  [unwired: 7 in]
            n16 = Append True/False String(1:w76, 2:"FAIL" ("真字符串"), 3:"PASS" ("真字符串")) -> (0:w77:string)  [unwired: 1 in]
            n17 = Build Array (concatenate)(w78, w72, w77) -> (w84:string[])
            n18 = Flatten To XML(anything=w84) -> (xml string=w83:string)
            n19 = call "AMC Send Local Message.vi"("Process (\"\" - local)"=w85, "Message Value"=w83, "Message Name"=w85) -> ()  [unwired: 7 in, 2 out]
          }
        }
        n20 = call <vilib>:"Space Constant.vi"() -> ("String"=w61:string)
        n21 = Concatenate Strings(w57, w61, w59) -> (w60:string)
        n22 = Bundle By Name(cluster=w63, "BEMF_Calibration.Read_ambient_temperature"=w54) -> (w62:T3)
        n23 = call "LogStatus.vi"("error in (no error)"=w53, "last message"=w64, "message"=w60) -> ("error  out"=w65:errorcluster)  [unwired: 8 in]
      }
      frame "5.2.1_4 Check Environment relative humidity value" {
        n24 = Unbundle By Name(w86) -> ("Table"=w90:string[][])  [unwired: 1 out]
        n25 = call "Select_Table_Vaule Enable_Disable.vi"("Action"=w91, "Table"=w90) -> ("Enable"=w92:bool)  [unwired: 8 in, 1 out]
        n26 = case shown="True" w92 {
          tunnel: ["Skip" ("response") w106] -> w93
          tunnel: w91 -> [_ w114]
          tunnel: w90 -> [_ w113]
          tunnel: [errorcluster {"status"=FALSE, "code"=0, "source"=""} ("错误输出") w105] -> w87
          tunnel: [-1 w104] -> w88
          frame False {
          }
          frame True {
            (unwired) "Read Environment Illuminance Value Success"
            w119 = "UIdisplay" ("Process (\"\" - local)")
            n27 = call "HD_Config.vi"("Step"=enum16{"Initial", "Write", "Read"}."Read") -> ("HD Config out"=w109:T5)  [unwired: 9 in, 1 out]
            n28 = Unbundle By Name(w109) -> ("Tempt&Hum.COM"=w107:refnum<visa-resource-name>)
            n29 = call "ADAM_Read.vi"("VISA resource name"=w107) -> ("error out"=w105:errorcluster, "humidity"=w104:dbl)  [unwired: 7 in, 2 out]
            n30 = Number To Fractional String(number=w104) -> (F-format string=w106:string)  [unwired: 3 in]
            n31 = call "Select_Table_Vaule.vi"("Vaule"=w106, "Action"=w114, "Table"=w113) -> ("Result"=w110:bool, "vaule"=w112:string[])  [unwired: 7 in]
            n32 = Append True/False String(1:w110, 2:"FAIL" ("真字符串"), 3:"PASS" ("真字符串")) -> (0:w111:string)  [unwired: 1 in]
            n33 = Build Array (concatenate)(w112, w106, w111) -> (w118:string[])
            n34 = Flatten To XML(anything=w118) -> (xml string=w117:string)
            n35 = call "AMC Send Local Message.vi"("Process (\"\" - local)"=w119, "Message Value"=w117, "Message Name"=w119) -> ()  [unwired: 7 in, 2 out]
          }
        }
        n36 = call <vilib>:"Space Constant.vi"() -> ("String"=w95:string)
        n37 = Concatenate Strings(w91, w95, w93) -> (w94:string)
        n38 = Bundle By Name(cluster=w97, "BEMF_Calibration.Read_ambient_temperature"=w88) -> (w96:T3)
        n39 = call "LogStatus.vi"("error in (no error)"=w87, "last message"=w98, "message"=w94) -> ("error  out"=w99:errorcluster)  [unwired: 8 in]
      }
      frame "5.2.1_5  Check Environment value from Lux sense" {
        n40 = Unbundle By Name(w120) -> ("Table"=w124:string[][])  [unwired: 1 out]
        n41 = call "Select_Table_Vaule Enable_Disable.vi"("Action"=w125, "Table"=w124) -> ("Enable"=w126:bool)  [unwired: 8 in, 1 out]
        n42 = case shown="True" w126 {
          tunnel: ["Skip" ("response") w139] -> w127
          tunnel: w125 -> [_ w145]
          tunnel: w124 -> [_ w144]
          tunnel: [errorcluster {"status"=FALSE, "code"=0, "source"=""} ("错误输出") w140] -> w121
          tunnel: [-1 0] -> w122
          frame False {
          }
          frame True {
            (unwired) "Read Environment Illuminance Value Success"
            w150 = "UIdisplay" ("Process (\"\" - local)")
            n43 = call "Read_Lux.vi"() -> ("error out"=w140:errorcluster, "Lux_Value"=w139:string)  [unwired: 9 in, 1 out]
            n44 = call "Select_Table_Vaule.vi"("Vaule"=w139, "Action"=w145, "Table"=w144) -> ("Result"=w141:bool, "vaule"=w143:string[])  [unwired: 7 in]
            n45 = Append True/False String(1:w141, 2:"FAIL" ("真字符串"), 3:"PASS" ("真字符串")) -> (0:w142:string)  [unwired: 1 in]
            n46 = Build Array (concatenate)(w143, w139, w142) -> (w149:string[])
            n47 = Flatten To XML(anything=w149) -> (xml string=w148:string)
            n48 = call "AMC Send Local Message.vi"("Process (\"\" - local)"=w150, "Message Value"=w148, "Message Name"=w150) -> ()  [unwired: 7 in, 2 out]
          }
        }
        n49 = call <vilib>:"Space Constant.vi"() -> ("String"=w129:string)
        n50 = Concatenate Strings(w125, w129, w127) -> (w128:string)
        n51 = Bundle By Name(cluster=w131, "BEMF_Calibration.Read_ambient_temperature"=w122) -> (w130:T3)
        n52 = call "LogStatus.vi"("error in (no error)"=w121, "last message"=w132, "message"=w128) -> ("error  out"=w133:errorcluster)  [unwired: 8 in]
      }
      frame "5.2.2_1 Make sure the USB type C connected to UUT" {
        n53 = Unbundle By Name(w153) -> ("Table"=w155:string[][])  [unwired: 1 out]
        n54 = call "Select_Table_Vaule Enable_Disable.vi"("Action"=w156, "Table"=w155) -> ("Enable"=w157:bool)  [unwired: 8 in, 1 out]
        n55 = case shown="True" w157 {
          tunnel: ["Skip" ("response") w170] -> w158
          tunnel: w156 -> [_ w176]
          tunnel: w155 -> [_ w175]
          tunnel: [errorcluster {"status"=FALSE, "code"=0, "source"=""} ("错误输出") _] -> _
          tunnel: [-1 0] -> w154
          frame False {
          }
          frame True {
            (unwired) "Read Environment Illuminance Value Success"
            w181 = "UIdisplay" ("Process (\"\" - local)")
            n56 = call "SendCmd.vi"("path"=path "C:/Users/user/Desktop/tool/5.bat") -> ("version info"=w170:string)  [unwired: 10 in]
            n57 = call "Select_Table_Vaule.vi"("Vaule"=w170, "Action"=w176, "Table"=w175) -> ("Result"=w172:bool, "vaule"=w174:string[])  [unwired: 7 in]
            n58 = Append True/False String(1:w172, 2:"FAIL" ("真字符串"), 3:"PASS" ("真字符串")) -> (0:w173:string)  [unwired: 1 in]
            n59 = Build Array (concatenate)(w174, w170, w173) -> (w180:string[])
            n60 = Flatten To XML(anything=w180) -> (xml string=w179:string)
            n61 = call "AMC Send Local Message.vi"("Process (\"\" - local)"=w181, "Message Value"=w179, "Message Name"=w181) -> ()  [unwired: 7 in, 2 out]
          }
        }
        n62 = call <vilib>:"Space Constant.vi"() -> ("String"=w160:string)
        n63 = Concatenate Strings(w156, w160, w158) -> (w159:string)
        n64 = Bundle By Name(cluster=w162, "BEMF_Calibration.Read_ambient_temperature"=w154) -> (w161:T3)
        n65 = call "LogStatus.vi"("error in (no error)"=w151, "last message"=w163, "message"=w159) -> ("error  out"=w164:errorcluster)  [unwired: 8 in]
      }
      frame "5.2.2_2 Verify Connection to UUT" {
        n66 = Unbundle By Name(w183) -> ("Table"=w186:string[][])  [unwired: 1 out]
        n67 = call "Select_Table_Vaule Enable_Disable.vi"("Action"=w187, "Table"=w186) -> ("Enable"=w188:bool)  [unwired: 8 in, 1 out]
        n68 = case shown="True" w188 {
          tunnel: ["Skip" ("response") w200] -> w189
          tunnel: w187 -> [_ w206]
          tunnel: w186 -> [_ w205]
          tunnel: [errorcluster {"status"=FALSE, "code"=0, "source"=""} ("错误输出") _] -> _
          tunnel: [-1 0] -> w184
          frame False {
          }
          frame True {
            (unwired) "Read Environment Illuminance Value Success"
            w211 = "UIdisplay" ("Process (\"\" - local)")
            n69 = call "SendCmd.vi"() -> ("version info"=w200:string)  [unwired: 11 in]
            n70 = call "Select_Table_Vaule.vi"("Vaule"=w200, "Action"=w206, "Table"=w205) -> ("Result"=w202:bool, "vaule"=w204:string[])  [unwired: 7 in]
            n71 = Append True/False String(1:w202, 2:"FAIL" ("真字符串"), 3:"PASS" ("真字符串")) -> (0:w203:string)  [unwired: 1 in]
            n72 = Build Array (concatenate)(w204, w200, w203) -> (w210:string[])
            n73 = Flatten To XML(anything=w210) -> (xml string=w209:string)
            n74 = call "AMC Send Local Message.vi"("Process (\"\" - local)"=w211, "Message Value"=w209, "Message Name"=w211) -> ()  [unwired: 7 in, 2 out]
          }
        }
        n75 = call <vilib>:"Space Constant.vi"() -> ("String"=w191:string)
        n76 = Concatenate Strings(w187, w191, w189) -> (w190:string)
        n77 = Bundle By Name(cluster=w193, "BEMF_Calibration.Read_ambient_temperature"=w184) -> (w192:T3)
        n78 = call "LogStatus.vi"("error in (no error)"=w182, "last message"=w194, "message"=w190) -> ("error  out"=w195:errorcluster)  [unwired: 8 in]
      }
      frame "5.2.2_3 Check Environment value from Lux sense" {
        n79 = Unbundle By Name(w212) -> ("Table"=w216:string[][])  [unwired: 1 out]
        n80 = call "Select_Table_Vaule Enable_Disable.vi"("Action"=w217, "Table"=w216) -> ("Enable"=w218:bool)  [unwired: 8 in, 1 out]
        n81 = case shown="True" w218 {
          tunnel: ["Skip" ("response") w231] -> w219
          tunnel: w217 -> [_ w237]
          tunnel: w216 -> [_ w236]
          tunnel: [errorcluster {"status"=FALSE, "code"=0, "source"=""} ("错误输出") w230] -> w213
          tunnel: [-1 0] -> w214
          frame False {
          }
          frame True {
            (unwired) "Read Environment Illuminance Value Success"
            w242 = "UIdisplay" ("Process (\"\" - local)")
            n82 = call "Read_Lux.vi"() -> ("error out"=w230:errorcluster, "Lux_Value"=w231:string)  [unwired: 9 in, 1 out]
            n83 = call "Select_Table_Vaule.vi"("Vaule"=w231, "Action"=w237, "Table"=w236) -> ("Result"=w233:bool, "vaule"=w235:string[])  [unwired: 7 in]
            n84 = Append True/False String(1:w233, 2:"FAIL" ("真字符串"), 3:"PASS" ("真字符串")) -> (0:w234:string)  [unwired: 1 in]
            n85 = Build Array (concatenate)(w235, w231, w234) -> (w241:string[])
            n86 = Flatten To XML(anything=w241) -> (xml string=w240:string)
            n87 = call "AMC Send Local Message.vi"("Process (\"\" - local)"=w242, "Message Value"=w240, "Message Name"=w242) -> ()  [unwired: 7 in, 2 out]
          }
        }
        n88 = call <vilib>:"Space Constant.vi"() -> ("String"=w221:string)
        n89 = Concatenate Strings(w217, w221, w219) -> (w220:string)
        n90 = Bundle By Name(cluster=w223, "BEMF_Calibration.Read_ambient_temperature"=w214) -> (w222:T3)
        n91 = call "LogStatus.vi"("error in (no error)"=w213, "last message"=w224, "message"=w220) -> ("error  out"=w225:errorcluster)  [unwired: 8 in]
      }
      frame "5.2.2_4 Start Test mode" {
        n92 = Unbundle By Name(w244) -> ("Table"=w247:string[][])  [unwired: 1 out]
        n93 = call "Select_Table_Vaule Enable_Disable.vi"("Action"=w248, "Table"=w247) -> ("Enable"=w249:bool)  [unwired: 8 in, 1 out]
        n94 = case shown="True" w249 {
          tunnel: ["Skip" ("response") w262] -> w250
          tunnel: w248 -> [_ w268]
          tunnel: w247 -> [_ w267]
          tunnel: [errorcluster {"status"=FALSE, "code"=0, "source"=""} ("错误输出") _] -> _
          tunnel: [-1 0] -> w245
          frame False {
          }
          frame True {
            (unwired) "Read Environment Illuminance Value Success"
            w273 = "UIdisplay" ("Process (\"\" - local)")
            n95 = call "SendCmd.vi"("path"=path "C:/Users/user/Desktop/tool/5.bat") -> ("version info"=w262:string)  [unwired: 10 in]
            n96 = call "Select_Table_Vaule.vi"("Vaule"=w262, "Action"=w268, "Table"=w267) -> ("Result"=w264:bool, "vaule"=w266:string[])  [unwired: 7 in]
            n97 = Append True/False String(1:w264, 2:"FAIL" ("真字符串"), 3:"PASS" ("真字符串")) -> (0:w265:string)  [unwired: 1 in]
            n98 = Build Array (concatenate)(w266, w262, w265) -> (w272:string[])
            n99 = Flatten To XML(anything=w272) -> (xml string=w271:string)
            n100 = call "AMC Send Local Message.vi"("Process (\"\" - local)"=w273, "Message Value"=w271, "Message Name"=w273) -> ()  [unwired: 7 in, 2 out]
          }
        }
        n101 = call <vilib>:"Space Constant.vi"() -> ("String"=w252:string)
        n102 = Concatenate Strings(w248, w252, w250) -> (w251:string)
        n103 = Bundle By Name(cluster=w254, "BEMF_Calibration.Read_ambient_temperature"=w245) -> (w253:T3)
        n104 = call "LogStatus.vi"("error in (no error)"=w243, "last message"=w255, "message"=w251) -> ("error  out"=w256:errorcluster)  [unwired: 8 in]
      }
      frame "5.2.2_5 Start camera test mode" {
        n105 = Unbundle By Name(w275) -> ("Table"=w278:string[][])  [unwired: 1 out]
        n106 = call "Select_Table_Vaule Enable_Disable.vi"("Action"=w279, "Table"=w278) -> ("Enable"=w280:bool)  [unwired: 8 in, 1 out]
        n107 = case shown="True" w280 {
          tunnel: ["Skip" ("response") w293] -> w281
          tunnel: w279 -> [_ w299]
          tunnel: w278 -> [_ w298]
          tunnel: [errorcluster {"status"=FALSE, "code"=0, "source"=""} ("错误输出") _] -> _
          tunnel: [-1 0] -> w276
          frame False {
          }
          frame True {
            (unwired) "Read Environment Illuminance Value Success"
            w304 = "UIdisplay" ("Process (\"\" - local)")
            n108 = call "SendCmd.vi"("path"=path "C:/Users/user/Desktop/tool/5.bat") -> ("version info"=w293:string)  [unwired: 10 in]
            n109 = call "Select_Table_Vaule.vi"("Vaule"=w293, "Action"=w299, "Table"=w298) -> ("Result"=w295:bool, "vaule"=w297:string[])  [unwired: 7 in]
            n110 = Append True/False String(1:w295, 2:"FAIL" ("真字符串"), 3:"PASS" ("真字符串")) -> (0:w296:string)  [unwired: 1 in]
            n111 = Build Array (concatenate)(w297, w293, w296) -> (w303:string[])
            n112 = Flatten To XML(anything=w303) -> (xml string=w302:string)
            n113 = call "AMC Send Local Message.vi"("Process (\"\" - local)"=w304, "Message Value"=w302, "Message Name"=w304) -> ()  [unwired: 7 in, 2 out]
          }
        }
        n114 = call <vilib>:"Space Constant.vi"() -> ("String"=w283:string)
        n115 = Concatenate Strings(w279, w283, w281) -> (w282:string)
        n116 = Bundle By Name(cluster=w285, "BEMF_Calibration.Read_ambient_temperature"=w276) -> (w284:T3)
        n117 = call "LogStatus.vi"("error in (no error)"=w274, "last message"=w286, "message"=w282) -> ("error  out"=w287:errorcluster)  [unwired: 8 in]
      }
      frame "5.2.2_6 get one RAW Image" {
        n118 = Unbundle By Name(w306) -> ("Table"=w309:string[][])  [unwired: 1 out]
        n119 = call "Select_Table_Vaule Enable_Disable.vi"("Action"=w310, "Table"=w309) -> ("Enable"=w311:bool)  [unwired: 8 in, 1 out]
        n120 = case shown="True" w311 {
          tunnel: ["Skip" ("response") w324] -> w312
          tunnel: w310 -> [_ w330]
          tunnel: w309 -> [_ w329]
          tunnel: [errorcluster {"status"=FALSE, "code"=0, "source"=""} ("错误输出") _] -> _
          tunnel: [-1 0] -> w307
          frame False {
          }
          frame True {
            (unwired) "Read Environment Illuminance Value Success"
            w335 = "UIdisplay" ("Process (\"\" - local)")
            n121 = call "SendCmd.vi"("path"=path "C:/Users/user/Desktop/tool/5.bat") -> ("version info"=w324:string)  [unwired: 10 in]
            n122 = call "Select_Table_Vaule.vi"("Vaule"=w324, "Action"=w330, "Table"=w329) -> ("Result"=w326:bool, "vaule"=w328:string[])  [unwired: 7 in]
            n123 = Append True/False String(1:w326, 2:"FAIL" ("真字符串"), 3:"PASS" ("真字符串")) -> (0:w327:string)  [unwired: 1 in]
            n124 = Build Array (concatenate)(w328, w324, w327) -> (w334:string[])
            n125 = Flatten To XML(anything=w334) -> (xml string=w333:string)
            n126 = call "AMC Send Local Message.vi"("Process (\"\" - local)"=w335, "Message Value"=w333, "Message Name"=w335) -> ()  [unwired: 7 in, 2 out]
          }
        }
        n127 = call <vilib>:"Space Constant.vi"() -> ("String"=w314:string)
        n128 = Concatenate Strings(w310, w314, w312) -> (w313:string)
        n129 = Bundle By Name(cluster=w316, "BEMF_Calibration.Read_ambient_temperature"=w307) -> (w315:T3)
        n130 = call "LogStatus.vi"("error in (no error)"=w305, "last message"=w317, "message"=w313) -> ("error  out"=w318:errorcluster)  [unwired: 8 in]
      }
      frame "5.2.2_7 Find Image  in the CLI tool directory" {
        n131 = Unbundle By Name(w337) -> ("Table"=w340:string[][])  [unwired: 1 out]
        n132 = call "Select_Table_Vaule Enable_Disable.vi"("Action"=w341, "Table"=w340) -> ("Enable"=w342:bool)  [unwired: 8 in, 1 out]
        n133 = case shown="True" w342 {
          tunnel: ["Skip" ("response") w355] -> w343
          tunnel: w341 -> [_ w361]
          tunnel: w340 -> [_ w360]
          tunnel: [errorcluster {"status"=FALSE, "code"=0, "source"=""} ("错误输出") _] -> _
          tunnel: [-1 0] -> w338
          frame False {
          }
          frame True {
            (unwired) "Read Environment Illuminance Value Success"
            w366 = "UIdisplay" ("Process (\"\" - local)")
            n134 = call "SendCmd.vi"("path"=path "C:/Users/user/Desktop/tool/5.bat") -> ("version info"=w355:string)  [unwired: 10 in]
            n135 = call "Select_Table_Vaule.vi"("Vaule"=w355, "Action"=w361, "Table"=w360) -> ("Result"=w357:bool, "vaule"=w359:string[])  [unwired: 7 in]
            n136 = Append True/False String(1:w357, 2:"FAIL" ("真字符串"), 3:"PASS" ("真字符串")) -> (0:w358:string)  [unwired: 1 in]
            n137 = Build Array (concatenate)(w359, w355, w358) -> (w365:string[])
            n138 = Flatten To XML(anything=w365) -> (xml string=w364:string)
            n139 = call "AMC Send Local Message.vi"("Process (\"\" - local)"=w366, "Message Value"=w364, "Message Name"=w366) -> ()  [unwired: 7 in, 2 out]
          }
        }
        n140 = call <vilib>:"Space Constant.vi"() -> ("String"=w345:string)
        n141 = Concatenate Strings(w341, w345, w343) -> (w344:string)
        n142 = Bundle By Name(cluster=w347, "BEMF_Calibration.Read_ambient_temperature"=w338) -> (w346:T3)
        n143 = call "LogStatus.vi"("error in (no error)"=w336, "last message"=w348, "message"=w344) -> ("error  out"=w349:errorcluster)  [unwired: 8 in]
      }
      frame "5.2.2_8 External software analyze raw image to generate calibration data" {
        n144 = Unbundle By Name(w368) -> ("Table"=w371:string[][])  [unwired: 1 out]
        n145 = call "Select_Table_Vaule Enable_Disable.vi"("Action"=w372, "Table"=w371) -> ("Enable"=w373:bool)  [unwired: 8 in, 1 out]
        n146 = case shown="True" w373 {
          tunnel: ["Skip" ("response") w385] -> w374
          tunnel: w372 -> [_ w391]
          tunnel: w371 -> [_ w390]
          tunnel: [errorcluster {"status"=FALSE, "code"=0, "source"=""} ("错误输出") _] -> _
          tunnel: [-1 0] -> w369
          frame False {
          }
          frame True {
            (unwired) "Read Environment Illuminance Value Success"
            w396 = "UIdisplay" ("Process (\"\" - local)")
            n147 = call "SendCmd.vi"() -> ("version info"=w385:string)  [unwired: 11 in]
            n148 = call "Select_Table_Vaule.vi"("Vaule"=w385, "Action"=w391, "Table"=w390) -> ("Result"=w387:bool, "vaule"=w389:string[])  [unwired: 7 in]
            n149 = Append True/False String(1:w387, 2:"FAIL" ("真字符串"), 3:"PASS" ("真字符串")) -> (0:w388:string)  [unwired: 1 in]
            n150 = Build Array (concatenate)(w389, w385, w388) -> (w395:string[])
            n151 = Flatten To XML(anything=w395) -> (xml string=w394:string)
            n152 = call "AMC Send Local Message.vi"("Process (\"\" - local)"=w396, "Message Value"=w394, "Message Name"=w396) -> ()  [unwired: 7 in, 2 out]
          }
        }
        n153 = call <vilib>:"Space Constant.vi"() -> ("String"=w376:string)
        n154 = Concatenate Strings(w372, w376, w374) -> (w375:string)
        n155 = Bundle By Name(cluster=w378, "BEMF_Calibration.Read_ambient_temperature"=w369) -> (w377:T3)
        n156 = call "LogStatus.vi"("error in (no error)"=w367, "last message"=w379, "message"=w375) -> ("error  out"=w380:errorcluster)  [unwired: 8 in]
      }
      frame "5.2.2_9 Write back calibration data to UUT" {
        n157 = Unbundle By Name(w398) -> ("Table"=w401:string[][])  [unwired: 1 out]
        n158 = call "Select_Table_Vaule Enable_Disable.vi"("Action"=w402, "Table"=w401) -> ("Enable"=w403:bool)  [unwired: 8 in, 1 out]
        n159 = case shown="True" w403 {
          tunnel: ["Skip" ("response") w415] -> w404
          tunnel: w402 -> [_ w421]
          tunnel: w401 -> [_ w420]
          tunnel: [errorcluster {"status"=FALSE, "code"=0, "source"=""} ("错误输出") _] -> _
          tunnel: [-1 0] -> w399
          frame False {
          }
          frame True {
            (unwired) "Read Environment Illuminance Value Success"
            w426 = "UIdisplay" ("Process (\"\" - local)")
            n160 = call "SendCmd.vi"() -> ("version info"=w415:string)  [unwired: 11 in]
            n161 = call "Select_Table_Vaule.vi"("Vaule"=w415, "Action"=w421, "Table"=w420) -> ("Result"=w417:bool, "vaule"=w419:string[])  [unwired: 7 in]
            n162 = Append True/False String(1:w417, 2:"FAIL" ("真字符串"), 3:"PASS" ("真字符串")) -> (0:w418:string)  [unwired: 1 in]
            n163 = Build Array (concatenate)(w419, w415, w418) -> (w425:string[])
            n164 = Flatten To XML(anything=w425) -> (xml string=w424:string)
            n165 = call "AMC Send Local Message.vi"("Process (\"\" - local)"=w426, "Message Value"=w424, "Message Name"=w426) -> ()  [unwired: 7 in, 2 out]
          }
        }
        n166 = call <vilib>:"Space Constant.vi"() -> ("String"=w406:string)
        n167 = Concatenate Strings(w402, w406, w404) -> (w405:string)
        n168 = Bundle By Name(cluster=w408, "BEMF_Calibration.Read_ambient_temperature"=w399) -> (w407:T3)
        n169 = call "LogStatus.vi"("error in (no error)"=w397, "last message"=w409, "message"=w405) -> ("error  out"=w410:errorcluster)  [unwired: 8 in]
      }
      frame "5.2.2_10 Start camera test mode" {
        n170 = Unbundle By Name(w428) -> ("Table"=w431:string[][])  [unwired: 1 out]
        n171 = call "Select_Table_Vaule Enable_Disable.vi"("Action"=w432, "Table"=w431) -> ("Enable"=w433:bool)  [unwired: 8 in, 1 out]
        n172 = case shown="True" w433 {
          tunnel: ["Skip" ("response") w445] -> w434
          tunnel: w432 -> [_ w451]
          tunnel: w431 -> [_ w450]
          tunnel: [errorcluster {"status"=FALSE, "code"=0, "source"=""} ("错误输出") _] -> _
          tunnel: [-1 0] -> w429
          frame False {
          }
          frame True {
            (unwired) "Read Environment Illuminance Value Success"
            w456 = "UIdisplay" ("Process (\"\" - local)")
            n173 = call "SendCmd.vi"() -> ("version info"=w445:string)  [unwired: 11 in]
            n174 = call "Select_Table_Vaule.vi"("Vaule"=w445, "Action"=w451, "Table"=w450) -> ("Result"=w447:bool, "vaule"=w449:string[])  [unwired: 7 in]
            n175 = Append True/False String(1:w447, 2:"FAIL" ("真字符串"), 3:"PASS" ("真字符串")) -> (0:w448:string)  [unwired: 1 in]
            n176 = Build Array (concatenate)(w449, w445, w448) -> (w455:string[])
            n177 = Flatten To XML(anything=w455) -> (xml string=w454:string)
            n178 = call "AMC Send Local Message.vi"("Process (\"\" - local)"=w456, "Message Value"=w454, "Message Name"=w456) -> ()  [unwired: 7 in, 2 out]
          }
        }
        n179 = call <vilib>:"Space Constant.vi"() -> ("String"=w436:string)
        n180 = Concatenate Strings(w432, w436, w434) -> (w435:string)
        n181 = Bundle By Name(cluster=w438, "BEMF_Calibration.Read_ambient_temperature"=w429) -> (w437:T3)
        n182 = call "LogStatus.vi"("error in (no error)"=w427, "last message"=w439, "message"=w435) -> ("error  out"=w440:errorcluster)  [unwired: 8 in]
      }
      frame "5.2.2_11 Stop Test Mode" {
        n183 = Unbundle By Name(w458) -> ("Table"=w461:string[][])  [unwired: 1 out]
        n184 = call "Select_Table_Vaule Enable_Disable.vi"("Action"=w462, "Table"=w461) -> ("Enable"=w463:bool)  [unwired: 8 in, 1 out]
        n185 = case shown="True" w463 {
          tunnel: ["Skip" ("response") w475] -> w464
          tunnel: w462 -> [_ w481]
          tunnel: w461 -> [_ w480]
          tunnel: [errorcluster {"status"=FALSE, "code"=0, "source"=""} ("错误输出") _] -> _
          tunnel: [-1 0] -> w459
          frame False {
          }
          frame True {
            (unwired) "Read Environment Illuminance Value Success"
            w486 = "UIdisplay" ("Process (\"\" - local)")
            n186 = call "SendCmd.vi"() -> ("version info"=w475:string)  [unwired: 11 in]
            n187 = call "Select_Table_Vaule.vi"("Vaule"=w475, "Action"=w481, "Table"=w480) -> ("Result"=w477:bool, "vaule"=w479:string[])  [unwired: 7 in]
            n188 = Append True/False String(1:w477, 2:"FAIL" ("真字符串"), 3:"PASS" ("真字符串")) -> (0:w478:string)  [unwired: 1 in]
            n189 = Build Array (concatenate)(w479, w475, w478) -> (w485:string[])
            n190 = Flatten To XML(anything=w485) -> (xml string=w484:string)
            n191 = call "AMC Send Local Message.vi"("Process (\"\" - local)"=w486, "Message Value"=w484, "Message Name"=w486) -> ()  [unwired: 7 in, 2 out]
          }
        }
        n192 = call <vilib>:"Space Constant.vi"() -> ("String"=w466:string)
        n193 = Concatenate Strings(w462, w466, w464) -> (w465:string)
        n194 = Bundle By Name(cluster=w468, "BEMF_Calibration.Read_ambient_temperature"=w459) -> (w467:T3)
        n195 = call "LogStatus.vi"("error in (no error)"=w457, "last message"=w469, "message"=w465) -> ("error  out"=w470:errorcluster)  [unwired: 8 in]
      }
      frame "5.2.2_12 Reboot UUT by EOL Test Command" {
        n196 = Unbundle By Name(w488) -> ("Table"=w491:string[][])  [unwired: 1 out]
        n197 = call "Select_Table_Vaule Enable_Disable.vi"("Action"=w492, "Table"=w491) -> ("Enable"=w493:bool)  [unwired: 8 in, 1 out]
        n198 = case shown="True" w493 {
          tunnel: ["Skip" ("response") w505] -> w494
          tunnel: w492 -> [_ w511]
          tunnel: w491 -> [_ w510]
          tunnel: [errorcluster {"status"=FALSE, "code"=0, "source"=""} ("错误输出") _] -> _
          tunnel: [-1 0] -> w489
          frame False {
          }
          frame True {
            (unwired) "Read Environment Illuminance Value Success"
            w516 = "UIdisplay" ("Process (\"\" - local)")
            n199 = call "SendCmd.vi"() -> ("version info"=w505:string)  [unwired: 11 in]
            n200 = call "Select_Table_Vaule.vi"("Vaule"=w505, "Action"=w511, "Table"=w510) -> ("Result"=w507:bool, "vaule"=w509:string[])  [unwired: 7 in]
            n201 = Append True/False String(1:w507, 2:"FAIL" ("真字符串"), 3:"PASS" ("真字符串")) -> (0:w508:string)  [unwired: 1 in]
            n202 = Build Array (concatenate)(w509, w505, w508) -> (w515:string[])
            n203 = Flatten To XML(anything=w515) -> (xml string=w514:string)
            n204 = call "AMC Send Local Message.vi"("Process (\"\" - local)"=w516, "Message Value"=w514, "Message Name"=w516) -> ()  [unwired: 7 in, 2 out]
          }
        }
        n205 = call <vilib>:"Space Constant.vi"() -> ("String"=w496:string)
        n206 = Concatenate Strings(w492, w496, w494) -> (w495:string)
        n207 = Bundle By Name(cluster=w498, "BEMF_Calibration.Read_ambient_temperature"=w489) -> (w497:T3)
        n208 = call "LogStatus.vi"("error in (no error)"=w487, "last message"=w499, "message"=w495) -> ("error  out"=w500:errorcluster)  [unwired: 8 in]
      }
      frame "5.2.2_13 Re-connect UUT by NFC" {
        n209 = Unbundle By Name(w518) -> ("Table"=w521:string[][])  [unwired: 1 out]
        n210 = call "Select_Table_Vaule Enable_Disable.vi"("Action"=w522, "Table"=w521) -> ("Enable"=w523:bool)  [unwired: 8 in, 1 out]
        n211 = case shown="True" w523 {
          tunnel: ["Skip" ("response") w535] -> w524
          tunnel: w522 -> [_ w541]
          tunnel: w521 -> [_ w540]
          tunnel: [errorcluster {"status"=FALSE, "code"=0, "source"=""} ("错误输出") _] -> _
          tunnel: [-1 0] -> w519
          frame False {
          }
          frame True {
            (unwired) "Read Environment Illuminance Value Success"
            w546 = "UIdisplay" ("Process (\"\" - local)")
            n212 = call "SendCmd.vi"() -> ("version info"=w535:string)  [unwired: 11 in]
            n213 = call "Select_Table_Vaule.vi"("Vaule"=w535, "Action"=w541, "Table"=w540) -> ("Result"=w537:bool, "vaule"=w539:string[])  [unwired: 7 in]
            n214 = Append True/False String(1:w537, 2:"FAIL" ("真字符串"), 3:"PASS" ("真字符串")) -> (0:w538:string)  [unwired: 1 in]
            n215 = Build Array (concatenate)(w539, w535, w538) -> (w545:string[])
            n216 = Flatten To XML(anything=w545) -> (xml string=w544:string)
            n217 = call "AMC Send Local Message.vi"("Process (\"\" - local)"=w546, "Message Value"=w544, "Message Name"=w546) -> ()  [unwired: 7 in, 2 out]
          }
        }
        n218 = call <vilib>:"Space Constant.vi"() -> ("String"=w526:string)
        n219 = Concatenate Strings(w522, w526, w524) -> (w525:string)
        n220 = Bundle By Name(cluster=w528, "BEMF_Calibration.Read_ambient_temperature"=w519) -> (w527:T3)
        n221 = call "LogStatus.vi"("error in (no error)"=w517, "last message"=w529, "message"=w525) -> ("error  out"=w530:errorcluster)  [unwired: 8 in]
      }
      frame "5.2.2_14 verify OBC setting by EOL Test command" {
        n222 = Unbundle By Name(w549) -> ("Table"=w552:string[][])  [unwired: 1 out]
        n223 = call "Select_Table_Vaule Enable_Disable.vi"("Action"=w553, "Table"=w552) -> ("Enable"=w554:bool)  [unwired: 8 in, 1 out]
        n224 = case shown="True" w554 {
          tunnel: ["Skip" ("response") w566] -> w555
          tunnel: w553 -> [_ w572]
          tunnel: w552 -> [_ w571]
          tunnel: [errorcluster {"status"=FALSE, "code"=0, "source"=""} ("错误输出") _] -> _
          tunnel: [-1 0] -> w550
          frame False {
          }
          frame True {
            (unwired) "Read Environment Illuminance Value Success"
            w577 = "UIdisplay" ("Process (\"\" - local)")
            n225 = call "SendCmd.vi"() -> ("version info"=w566:string)  [unwired: 11 in]
            n226 = call "Select_Table_Vaule.vi"("Vaule"=w566, "Action"=w572, "Table"=w571) -> ("Result"=w568:bool, "vaule"=w570:string[])  [unwired: 7 in]
            n227 = Append True/False String(1:w568, 2:"FAIL" ("真字符串"), 3:"PASS" ("真字符串")) -> (0:w569:string)  [unwired: 1 in]
            n228 = Build Array (concatenate)(w570, w566, w569) -> (w576:string[])
            n229 = Flatten To XML(anything=w576) -> (xml string=w575:string)
            n230 = call "AMC Send Local Message.vi"("Process (\"\" - local)"=w577, "Message Value"=w575, "Message Name"=w577) -> ()  [unwired: 7 in, 2 out]
          }
        }
        n231 = call <vilib>:"Space Constant.vi"() -> ("String"=w557:string)
        n232 = Concatenate Strings(w553, w557, w555) -> (w556:string)
        n233 = Bundle By Name(cluster=w559, "BEMF_Calibration.Read_ambient_temperature"=w550) -> (w558:T3)
        n234 = call "LogStatus.vi"("error in (no error)"=w547, "last message"=w560, "message"=w556) -> ("error  out"=w561:errorcluster)  [unwired: 8 in]
      }
      frame "Start Test mode" {
        n235 = Unbundle By Name(w580) -> ("Table"=w582:string[][])
        n236 = call "Select_Table_Vaule Enable_Disable.vi"("Action"=w585, "Table"=w582) -> ("Enable"=w586:bool)  [unwired: 8 in, 1 out]
        n237 = case shown="True" w586 {
          tunnel: ["Skip" ("response") w597] -> w583
          tunnel: w585 -> [_ w598]
          tunnel: w582 -> [_ w602]
          frame False {
          }
          frame True {
            w607 = "UIdisplay" ("Process (\"\" - local)")
            n238 = call "SendCmd.vi"("path"=path "C:/Users/user/Desktop/tool/5.bat") -> ("version info"=w597:string)  [unwired: 10 in]
            n239 = call "Select_Table_Vaule.vi"("Vaule"=w597, "Action"=w598, "Table"=w602) -> ("Result"=w600:bool, "vaule"=w601:string[])  [unwired: 7 in]
            n240 = Append True/False String(1:w600, 2:"FAIL" ("真字符串"), 3:"PASS" ("真字符串")) -> (0:w599:string)  [unwired: 1 in]
            n241 = Build Array (concatenate)(w601, w597, w599) -> (w606:string[])
            n242 = Flatten To XML(anything=w606) -> (xml string=w605:string)
            n243 = call "AMC Send Local Message.vi"("Process (\"\" - local)"=w607, "Message Value"=w605, "Message Name"=w607) -> ()  [unwired: 7 in, 2 out]
          }
        }
        n244 = call <vilib>:"Space Constant.vi"() -> ("String"=w588:string)
        n245 = Concatenate Strings(w585, w588, w583) -> (w587:string)
        n246 = case shown="No Error" w578 {
          tunnel: [_ TRUE] -> w584
          tunnel: ["Start camera test mode" "Error"] -> w579
          frame No Error {
          }
          frame Error {
          }
        }
        n247 = call "LogStatus.vi"("error in (no error)"=w578, "last message"=w589, "message"=w587) -> ("error  out"=w590:errorcluster)  [unwired: 8 in]
      }
      frame "get one RAW Image" {
        n248 = Unbundle By Name(w609) -> ("Table"=w612:string[][])
        n249 = call "Select_Table_Vaule Enable_Disable.vi"("Action"=w615, "Table"=w612) -> ("Enable"=w616:bool)  [unwired: 8 in, 1 out]
        n250 = case shown="True" w616 {
          tunnel: ["Skip" ("response") w628] -> w613
          tunnel: w615 -> [_ w626]
          tunnel: w612 -> [_ w639]
          tunnel: [_ w632] -> w610
          frame False {
          }
          frame True {
            w644 = "UIdisplay" ("Process (\"\" - local)")
            n251 = Unbundle By Name(T6 {"getVersion"="682_eol_cli.exe -f version -t 0", "Start Test mode"="682_eol_cli.exe -f test -p 1", "Start camera test mode P1"="682_eol_cli.exe -f camera -p 1", "get one RAW Image"="“682_eol_cli.exe -f camera -p 2", "Start camera test mode P0"="682_eol_cli.exe -f camera -p 0", "Stop Test Mode"="682_eol_cli.exe -f test -p 0", "Stop Camera"="682_eol_cli.exe -f camera -p 0"} ("输入簇")) -> ("get one RAW Image"=w635:string)
            n252 = call "SendCmd.vi"(9:w635, "path"="D:\\Program Files\\MVTec\\HALCON-17.12-Progress\\bin\\x64-win64\\hdevelop.exe" ("exe")) -> (0:w632, "version info"=w629:string, 2:w630, 3:w627)  [unwired: 6 in]
            n253 = Equal To 0?(x=w630) -> (x = 0?=w631:bool)
            n254 = case shown="True" w631 {
              tunnel: w629 -> [_ w646]
              tunnel: [w645 w646] -> w628
              tunnel: w627 -> [w645 _]
              frame False {
              }
              frame True {
              }
            }
            n255 = call "Select_Table_Vaule.vi"("Vaule"=w628, "Action"=w626, "Table"=w639) -> ("Result"=w637:bool, "vaule"=w638:string[])  [unwired: 7 in]
            n256 = Append True/False String(1:w637, 2:"FAIL" ("真字符串"), 3:"PASS" ("真字符串")) -> (0:w636:string)  [unwired: 1 in]
            n257 = Build Array (concatenate)(w638, w628, w636) -> (w643:string[])
            n258 = Flatten To XML(anything=w643) -> (xml string=w642:string)
            n259 = call "AMC Send Local Message.vi"("Process (\"\" - local)"=w644, "Message Value"=w642, "Message Name"=w644) -> ()  [unwired: 7 in, 2 out]
          }
        }
        n260 = call <vilib>:"Space Constant.vi"() -> ("String"=w618:string)
        n261 = Concatenate Strings(w615, w618, w613) -> (w617:string)
        n262 = case shown="No Error" w610 {
          tunnel: [_ TRUE] -> w614
          tunnel: ["Check  Image Is Exist" "Error"] -> w608
          frame No Error {
          }
          frame Error {
          }
        }
        n263 = call "LogStatus.vi"("error in (no error)"=w610, "last message"=w619, "message"=w617) -> ("error  out"=w620:errorcluster)  [unwired: 8 in]
      }
      frame "Check  Image Is Exist" {
        n264 = Unbundle By Name(w648) -> ("Table"=w651:string[][])
        n265 = call "Select_Table_Vaule Enable_Disable.vi"("Action"=w654, "Table"=w651) -> ("Enable"=w655:bool)  [unwired: 8 in, 1 out]
        n266 = case shown="True" w655 {
          tunnel: ["Skip" ("response") w665] -> w652
          tunnel: w654 -> [_ w669]
          tunnel: w651 -> [_ w673]
          tunnel: [_ w667] -> w649
          frame False {
          }
          frame True {
            w678 = "UIdisplay" ("Process (\"\" - local)")
            n267 = call <vilib>:"Check if File or Folder Exists.vi"("path"="Image path") -> ("error out"=w667:errorcluster, "file or folder exists?"=w666:bool)  [unwired: 8 in, 1 out]
            n268 = case shown="False" w666 {
              tunnel: ["Image Save Fail" "Image Save Success"] -> w665
              frame False {
              }
              frame True {
              }
            }
            n269 = call "Select_Table_Vaule.vi"("Vaule"=w665, "Action"=w669, "Table"=w673) -> ("Result"=w671:bool, "vaule"=w672:string[])  [unwired: 7 in]
            n270 = Append True/False String(1:w671, 2:"FAIL" ("真字符串"), 3:"PASS" ("真字符串")) -> (0:w670:string)  [unwired: 1 in]
            n271 = Build Array (concatenate)(w672, w665, w670) -> (w677:string[])
            n272 = Flatten To XML(anything=w677) -> (xml string=w676:string)
            n273 = call "AMC Send Local Message.vi"("Process (\"\" - local)"=w678, "Message Value"=w676, "Message Name"=w678) -> ()  [unwired: 7 in, 2 out]
          }
        }
        n274 = call <vilib>:"Space Constant.vi"() -> ("String"=w657:string)
        n275 = Concatenate Strings(w654, w657, w652) -> (w656:string)
        n276 = case shown="No Error" w649 {
          tunnel: [_ TRUE] -> w653
          tunnel: ["External software analyze image to generate calibration data " "Error"] -> w647
          frame No Error {
          }
          frame Error {
          }
        }
        n277 = call "LogStatus.vi"("error in (no error)"=w649, "last message"=w658, "message"=w656) -> ("error  out"=w659:errorcluster)  [unwired: 8 in]
      }
      frame "External software analyze image to generate calibration data" {
        # "Write back  calibration data"
        n278 = Unbundle By Name(w682) -> ("Table"=w685:string[][])
        n279 = call "Select_Table_Vaule Enable_Disable.vi"("Action"=w688, "Table"=w685) -> ("Enable"=w689:bool)  [unwired: 8 in, 1 out]
        n280 = case shown="True" w689 {
          tunnel: ["Skip" ("response") w704] -> w686
          tunnel: w688 -> [_ w702]
          tunnel: w685 -> [_ w708]
          tunnel: [_ w701] -> w683
          frame False {
          }
          frame True {
            w713 = "UIdisplay" ("Process (\"\" - local)")
            # "第三方软件的路径与调用"
            n281 = call "SendCmd.vi"("path"="D:\\Program Files\\MVTec\\HALCON-17.12-Progress\\bin\\x64-win64\\hdevelop.exe" ("exe")) -> (0:w701, 2:w700)  [unwired: 8 in, 1 out]
            n282 = Equal To 0?(x=w700) -> (x = 0?=w699:bool)
            n283 = case shown="False" w699 {
              tunnel: ["Generate Image calibration data Fail" "Generate Image calibration data Success"] -> w704
              frame False {
              }
              frame True {
              }
            }
            n284 = call "Select_Table_Vaule.vi"("Vaule"=w704, "Action"=w702, "Table"=w708) -> ("Result"=w706:bool, "vaule"=w707:string[])  [unwired: 7 in]
            n285 = Append True/False String(1:w706, 2:"FAIL" ("真字符串"), 3:"PASS" ("真字符串")) -> (0:w705:string)  [unwired: 1 in]
            n286 = Build Array (concatenate)(w707, w704, w705) -> (w712:string[])
            n287 = Flatten To XML(anything=w712) -> (xml string=w711:string)
            n288 = call "AMC Send Local Message.vi"("Process (\"\" - local)"=w713, "Message Value"=w711, "Message Name"=w713) -> ()  [unwired: 7 in, 2 out]
          }
        }
        n289 = call <vilib>:"Space Constant.vi"() -> ("String"=w691:string)
        n290 = Concatenate Strings(w688, w691, w686) -> (w690:string)
        n291 = case shown="No Error" w683 {
          tunnel: [_ TRUE] -> w687
          tunnel: ["Write back  calibration data" "Error"] -> w681
          frame No Error {
          }
          frame Error {
          }
        }
        n292 = call "LogStatus.vi"("error in (no error)"=w683, "last message"=w692, "message"=w690) -> ("error  out"=w693:errorcluster)  [unwired: 8 in]
      }
      frame "Write back  calibration data" {
        # "Write back  calibration data"
        n293 = Unbundle By Name(w717) -> ("Table"=w720:string[][])
        n294 = call "Select_Table_Vaule Enable_Disable.vi"("Action"=w723, "Table"=w720) -> ("Enable"=w724:bool)  [unwired: 8 in, 1 out]
        n295 = case shown="True" w724 {
          tunnel: ["Skip" ("response") w738] -> w721
          tunnel: w723 -> [_ w739]
          tunnel: w720 -> [_ w743]
          tunnel: [_ w734] -> w718
          frame False {
          }
          frame True {
            w748 = "UIdisplay" ("Process (\"\" - local)")
            # "第三方软件的路径与调用"
            # "Write back “ calibration data” to UUT Success"
            n296 = call "SendCmd.vi"("path"="D:\\Program Files\\MVTec\\HALCON-17.12-Progress\\bin\\x64-win64\\hdevelop.exe" ("exe")) -> (0:w734, 2:w736)  [unwired: 8 in, 1 out]
            n297 = Equal To 0?(x=w736) -> (x = 0?=w735:bool)
            n298 = case shown="False" w735 {
              tunnel: ["Write back “ calibration data” to UUT Fail" "Write back “ calibration data” to UUT Success"] -> w738
              frame False {
              }
              frame True {
              }
            }
            n299 = call "Select_Table_Vaule.vi"("Vaule"=w738, "Action"=w739, "Table"=w743) -> ("Result"=w741:bool, "vaule"=w742:string[])  [unwired: 7 in]
            n300 = Append True/False String(1:w741, 2:"FAIL" ("真字符串"), 3:"PASS" ("真字符串")) -> (0:w740:string)  [unwired: 1 in]
            n301 = Build Array (concatenate)(w742, w738, w740) -> (w747:string[])
            n302 = Flatten To XML(anything=w747) -> (xml string=w746:string)
            n303 = call "AMC Send Local Message.vi"("Process (\"\" - local)"=w748, "Message Value"=w746, "Message Name"=w748) -> ()  [unwired: 7 in, 2 out]
          }
        }
        n304 = call <vilib>:"Space Constant.vi"() -> ("String"=w726:string)
        n305 = Concatenate Strings(w723, w726, w721) -> (w725:string)
        n306 = case shown="No Error" w718 {
          tunnel: [_ TRUE] -> w722
          tunnel: ["Start camera test modeP0" "Error"] -> w716
          frame No Error {
          }
          frame Error {
          }
        }
        n307 = call "LogStatus.vi"("error in (no error)"=w718, "last message"=w727, "message"=w725) -> ("error  out"=w728:errorcluster)  [unwired: 8 in]
      }
      frame "Start camera test modeP0" {
        # "Write back  calibration data"
        n308 = Unbundle By Name(w752) -> ("Table"=w755:string[][])
        n309 = call "Select_Table_Vaule Enable_Disable.vi"("Action"=w758, "Table"=w755) -> ("Enable"=w759:bool)  [unwired: 8 in, 1 out]
        n310 = case shown="True" w759 {
          tunnel: ["Skip" ("response") w770] -> w756
          tunnel: w758 -> [_ w778]
          tunnel: w755 -> [_ w782]
          tunnel: [_ w769] -> w753
          frame False {
          }
          frame True {
            w787 = "UIdisplay" ("Process (\"\" - local)")
            # "第三方软件的路径与调用"
            n311 = Unbundle By Name(T6 {"getVersion"="682_eol_cli.exe -f version -t 0", "Start Test mode"="682_eol_cli.exe -f test -p 1", "Start camera test mode P1"="682_eol_cli.exe -f camera -p 1", "get one RAW Image"="“682_eol_cli.exe -f camera -p 2", "Start camera test mode P0"="682_eol_cli.exe -f camera -p 0", "Stop Test Mode"="682_eol_cli.exe -f test -p 0", "Stop Camera"="682_eol_cli.exe -f camera -p 0"} ("输入簇")) -> ("Start camera test mode P0"=w777:string)
            n312 = call "SendCmd.vi"(9:w777, "path"="D:\\Program Files\\MVTec\\HALCON-17.12-Progress\\bin\\x64-win64\\hdevelop.exe" ("exe")) -> (0:w769, "version info"=w772:string, 2:w773, 3:w771)  [unwired: 6 in]
            n313 = Equal To 0?(x=w773) -> (x = 0?=w774:bool)
            n314 = case shown="False" w774 {
              tunnel: w772 -> [_ w789]
              tunnel: [w788 w789] -> w770
              tunnel: w771 -> [w788 _]
              frame False {
              }
              frame True {
              }
            }
            n315 = call "Select_Table_Vaule.vi"("Vaule"=w770, "Action"=w778, "Table"=w782) -> ("Result"=w780:bool, "vaule"=w781:string[])  [unwired: 7 in]
            n316 = Append True/False String(1:w780, 2:"FAIL" ("真字符串"), 3:"PASS" ("真字符串")) -> (0:w779:string)  [unwired: 1 in]
            n317 = Build Array (concatenate)(w781, w770, w779) -> (w786:string[])
            n318 = Flatten To XML(anything=w786) -> (xml string=w785:string)
            n319 = call "AMC Send Local Message.vi"("Process (\"\" - local)"=w787, "Message Value"=w785, "Message Name"=w787) -> ()  [unwired: 7 in, 2 out]
          }
        }
        n320 = call <vilib>:"Space Constant.vi"() -> ("String"=w761:string)
        n321 = Concatenate Strings(w758, w761, w756) -> (w760:string)
        n322 = case shown="No Error" w753 {
          tunnel: [_ TRUE] -> w757
          tunnel: ["Stop Test Mode" "Error"] -> w751
          frame No Error {
          }
          frame Error {
          }
        }
        n323 = call "LogStatus.vi"("error in (no error)"=w753, "last message"=w762, "message"=w760) -> ("error  out"=w763:errorcluster)  [unwired: 8 in]
      }
      frame "Stop Test Mode" {
        # "Write back  calibration data"
        n324 = Unbundle By Name(w791) -> ("Table"=w794:string[][])
        n325 = call "Select_Table_Vaule Enable_Disable.vi"("Action"=w797, "Table"=w794) -> ("Enable"=w798:bool)  [unwired: 8 in, 1 out]
        n326 = case shown="True" w798 {
          tunnel: ["Skip" ("response") w809] -> w795
          tunnel: w797 -> [_ w817]
          tunnel: w794 -> [_ w821]
          tunnel: [_ w808] -> w792
          frame False {
          }
          frame True {
            w826 = "UIdisplay" ("Process (\"\" - local)")
            # "第三方软件的路径与调用"
            n327 = Unbundle By Name(T6 {"getVersion"="682_eol_cli.exe -f version -t 0", "Start Test mode"="682_eol_cli.exe -f test -p 1", "Start camera test mode P1"="682_eol_cli.exe -f camera -p 1", "get one RAW Image"="“682_eol_cli.exe -f camera -p 2", "Start camera test mode P0"="682_eol_cli.exe -f camera -p 0", "Stop Test Mode"="682_eol_cli.exe -f test -p 0", "Stop Camera"="682_eol_cli.exe -f camera -p 0"} ("输入簇")) -> ("Stop Test Mode"=w816:string)
            n328 = call "SendCmd.vi"(9:w816, "path"="D:\\Program Files\\MVTec\\HALCON-17.12-Progress\\bin\\x64-win64\\hdevelop.exe" ("exe")) -> (0:w808, "version info"=w811:string, 2:w812, 3:w810)  [unwired: 6 in]
            n329 = Equal To 0?(x=w812) -> (x = 0?=w813:bool)
            n330 = case shown="False" w813 {
              tunnel: w811 -> [_ w828]
              tunnel: [w827 w828] -> w809
              tunnel: w810 -> [w827 _]
              frame False {
              }
              frame True {
              }
            }
            n331 = call "Select_Table_Vaule.vi"("Vaule"=w809, "Action"=w817, "Table"=w821) -> ("Result"=w819:bool, "vaule"=w820:string[])  [unwired: 7 in]
            n332 = Append True/False String(1:w819, 2:"FAIL" ("真字符串"), 3:"PASS" ("真字符串")) -> (0:w818:string)  [unwired: 1 in]
            n333 = Build Array (concatenate)(w820, w809, w818) -> (w825:string[])
            n334 = Flatten To XML(anything=w825) -> (xml string=w824:string)
            n335 = call "AMC Send Local Message.vi"("Process (\"\" - local)"=w826, "Message Value"=w824, "Message Name"=w826) -> ()  [unwired: 7 in, 2 out]
          }
        }
        n336 = call <vilib>:"Space Constant.vi"() -> ("String"=w800:string)
        n337 = Concatenate Strings(w797, w800, w795) -> (w799:string)
        n338 = case shown="No Error" w792 {
          tunnel: [_ TRUE] -> w796
          tunnel: ["Reboot UUT" "Error"] -> w790
          frame No Error {
          }
          frame Error {
          }
        }
        n339 = call "LogStatus.vi"("error in (no error)"=w792, "last message"=w801, "message"=w799) -> ("error  out"=w802:errorcluster)  [unwired: 8 in]
      }
      frame "Reboot UUT" {
        # "Re-connect UUT and verify connection to UUT"
        # "这部分程序目前待定，不确定是否需要"
        # "Write back  calibration data"
        n340 = Unbundle By Name(w830) -> ("Table"=w833:string[][])
        n341 = call "Select_Table_Vaule Enable_Disable.vi"("Action"=w836, "Table"=w833) -> ("Enable"=w837:bool)  [unwired: 8 in, 1 out]
        n342 = case shown="True" w837 {
          tunnel: ["Skip" ("response") w848] -> w834
          tunnel: w836 -> [_ w856]
          tunnel: w833 -> [_ w860]
          tunnel: [_ w847] -> w831
          frame False {
          }
          frame True {
            w865 = "UIdisplay" ("Process (\"\" - local)")
            # "第三方软件的路径与调用"
            n343 = Unbundle By Name(T6 {"getVersion"="682_eol_cli.exe -f version -t 0", "Start Test mode"="682_eol_cli.exe -f test -p 1", "Start camera test mode P1"="682_eol_cli.exe -f camera -p 1", "get one RAW Image"="“682_eol_cli.exe -f camera -p 2", "Start camera test mode P0"="682_eol_cli.exe -f camera -p 0", "Stop Test Mode"="682_eol_cli.exe -f test -p 0", "Stop Camera"="682_eol_cli.exe -f camera -p 0"} ("输入簇")) -> ("Stop Test Mode"=w855:string)
            n344 = call "SendCmd.vi"(9:w855, "path"="D:\\Program Files\\MVTec\\HALCON-17.12-Progress\\bin\\x64-win64\\hdevelop.exe" ("exe")) -> (0:w847, "version info"=w850:string, 2:w851, 3:w849)  [unwired: 6 in]
            n345 = Equal To 0?(x=w851) -> (x = 0?=w852:bool)
            n346 = case shown="False" w852 {
              tunnel: w850 -> [_ w867]
              tunnel: [w866 w867] -> w848
              tunnel: w849 -> [w866 _]
              frame False {
              }
              frame True {
              }
            }
            n347 = call "Select_Table_Vaule.vi"("Vaule"=w848, "Action"=w856, "Table"=w860) -> ("Result"=w858:bool, "vaule"=w859:string[])  [unwired: 7 in]
            n348 = Append True/False String(1:w858, 2:"FAIL" ("真字符串"), 3:"PASS" ("真字符串")) -> (0:w857:string)  [unwired: 1 in]
            n349 = Build Array (concatenate)(w859, w848, w857) -> (w864:string[])
            n350 = Flatten To XML(anything=w864) -> (xml string=w863:string)
            n351 = call "AMC Send Local Message.vi"("Process (\"\" - local)"=w865, "Message Value"=w863, "Message Name"=w865) -> ()  [unwired: 7 in, 2 out]
          }
        }
        n352 = call <vilib>:"Space Constant.vi"() -> ("String"=w839:string)
        n353 = Concatenate Strings(w836, w839, w834) -> (w838:string)
        n354 = case shown="No Error" w831 {
          tunnel: [_ TRUE] -> w835
          tunnel: ["Re-connect UUT and verify connection to UUT" "Error"] -> w829
          frame No Error {
          }
          frame Error {
          }
        }
        n355 = call "LogStatus.vi"("error in (no error)"=w831, "last message"=w840, "message"=w838) -> ("error  out"=w841:errorcluster)  [unwired: 8 in]
      }
      frame "Re-connect UUT and verify connection to UUT" {
        # "Write back  calibration data"
        n356 = Unbundle By Name(w869) -> ("Table"=w872:string[][])
        n357 = call "Select_Table_Vaule Enable_Disable.vi"("Action"=w875, "Table"=w872) -> ("Enable"=w876:bool)  [unwired: 8 in, 1 out]
        n358 = case shown="True" w876 {
          tunnel: ["Skip" ("response") w887] -> w873
          tunnel: w875 -> [_ w895]
          tunnel: w872 -> [_ w899]
          tunnel: [_ w886] -> w870
          frame False {
          }
          frame True {
            w904 = "UIdisplay" ("Process (\"\" - local)")
            # "重新连接"
            n359 = Unbundle By Name(T6 {"getVersion"="682_eol_cli.exe -f version -t 0", "Start Test mode"="682_eol_cli.exe -f test -p 1", "Start camera test mode P1"="682_eol_cli.exe -f camera -p 1", "get one RAW Image"="“682_eol_cli.exe -f camera -p 2", "Start camera test mode P0"="682_eol_cli.exe -f camera -p 0", "Stop Test Mode"="682_eol_cli.exe -f test -p 0", "Stop Camera"="682_eol_cli.exe -f camera -p 0"} ("输入簇")) -> ("getVersion"=w894:string)
            n360 = call "SendCmd.vi"(9:w894, "path"="D:\\Program Files\\MVTec\\HALCON-17.12-Progress\\bin\\x64-win64\\hdevelop.exe" ("exe")) -> (0:w886, "version info"=w889:string, 2:w890, 3:w888)  [unwired: 6 in]
            n361 = Equal To 0?(x=w890) -> (x = 0?=w891:bool)
            n362 = case shown="True" w891 {
              tunnel: w889 -> [_ w906]
              tunnel: [w905 w906] -> w887
              tunnel: w888 -> [w905 _]
              frame False {
                (unwired) "Error：UUT Reconnected NFC fail !"
              }
              frame True {
                (unwired) "UUT Reconnection NFC successful"
              }
            }
            n363 = call "Select_Table_Vaule.vi"("Vaule"=w887, "Action"=w895, "Table"=w899) -> ("Result"=w897:bool, "vaule"=w898:string[])  [unwired: 7 in]
            n364 = Append True/False String(1:w897, 2:"FAIL" ("真字符串"), 3:"PASS" ("真字符串")) -> (0:w896:string)  [unwired: 1 in]
            n365 = Build Array (concatenate)(w898, w887, w896) -> (w903:string[])
            n366 = Flatten To XML(anything=w903) -> (xml string=w902:string)
            n367 = call "AMC Send Local Message.vi"("Process (\"\" - local)"=w904, "Message Value"=w902, "Message Name"=w904) -> ()  [unwired: 7 in, 2 out]
          }
        }
        n368 = call <vilib>:"Space Constant.vi"() -> ("String"=w878:string)
        n369 = Concatenate Strings(w875, w878, w873) -> (w877:string)
        n370 = case shown="No Error" w870 {
          tunnel: [_ TRUE] -> w874
          tunnel: ["To verify OBC setting" "Error"] -> w868
          frame No Error {
          }
          frame Error {
          }
        }
        n371 = call "LogStatus.vi"("error in (no error)"=w870, "last message"=w879, "message"=w877) -> ("error  out"=w880:errorcluster)  [unwired: 8 in]
      }
      frame "To verify OBC setting" {
        # "这部分代码待定"
        # "Write back  calibration data"
        n372 = Unbundle By Name(w908) -> ("Table"=w911:string[][])
        n373 = call "Select_Table_Vaule Enable_Disable.vi"("Action"=w914, "Table"=w911) -> ("Enable"=w915:bool)  [unwired: 8 in, 1 out]
        n374 = case shown="True" w915 {
          tunnel: ["Skip" ("response") w927] -> w912
          tunnel: w914 -> [_ w935]
          tunnel: w911 -> [_ w938]
          tunnel: [_ w926] -> w909
          frame False {
          }
          frame True {
            w943 = "UIdisplay" ("Process (\"\" - local)")
            n375 = Unbundle By Name(T6 {"getVersion"="682_eol_cli.exe -f version -t 0", "Start Test mode"="682_eol_cli.exe -f test -p 1", "Start camera test mode P1"="682_eol_cli.exe -f camera -p 1", "get one RAW Image"="“682_eol_cli.exe -f camera -p 2", "Start camera test mode P0"="682_eol_cli.exe -f camera -p 0", "Stop Test Mode"="682_eol_cli.exe -f test -p 0", "Stop Camera"="682_eol_cli.exe -f camera -p 0"} ("输入簇")) -> ("getVersion"=w934:string)
            n376 = call "SendCmd.vi"(9:w934, "path"="D:\\Program Files\\MVTec\\HALCON-17.12-Progress\\bin\\x64-win64\\hdevelop.exe" ("exe")) -> (0:w926, "version info"=w929:string, 2:w930, 3:w928)  [unwired: 6 in]
            n377 = Equal To 0?(x=w930) -> (x = 0?=w931:bool)
            n378 = case shown="True" w931 {
              tunnel: w929 -> [_ w945]
              tunnel: [w944 w945] -> w927
              tunnel: w928 -> [w944 _]
              frame False {
                (unwired) "Error：UUT Reconnected NFC fail !"
              }
              frame True {
                (unwired) "UUT Reconnection NFC successful"
              }
            }
            n379 = call "Select_Table_Vaule.vi"("Vaule"=w927, "Action"=w935, "Table"=w938) -> ("Result"=w925:bool, "vaule"=w937:string[])  [unwired: 7 in]
            n380 = Append True/False String(1:w925, 2:"FAIL" ("真字符串"), 3:"PASS" ("真字符串")) -> (0:w936:string)  [unwired: 1 in]
            n381 = Build Array (concatenate)(w937, w927, w936) -> (w942:string[])
            n382 = Flatten To XML(anything=w942) -> (xml string=w941:string)
            n383 = call "AMC Send Local Message.vi"("Process (\"\" - local)"=w943, "Message Value"=w941, "Message Name"=w943) -> ()  [unwired: 7 in, 2 out]
          }
        }
        n384 = call <vilib>:"Space Constant.vi"() -> ("String"=w917:string)
        n385 = Concatenate Strings(w914, w917, w912) -> (w916:string)
        n386 = case shown="No Error" w909 {
          tunnel: [_ TRUE] -> w913
          tunnel: ["To verify OBC setting" "Error"] -> w907
          frame No Error {
          }
          frame Error {
          }
        }
        n387 = call "LogStatus.vi"("error in (no error)"=w909, "last message"=w918, "message"=w916) -> ("error  out"=w919:errorcluster)  [unwired: 8 in]
      }
      frame "Calibration_Read_and_check_Calibration_value_A" {
        n388 = Unbundle By Name(w986) -> ("Table"=w996:string[][], "daemon reference"=w1003:refnum<k5>, "Config"=w994:string[][])
        n389 = Unbundle By Name(w974) -> ("MES bool"=w977:refnum<vi>)
        n390 = call "HD_Config.vi"("Step"=enum16{"Initial", "Write", "Read"}."Read") -> ("HD Config out"=w976:T5)  [unwired: 9 in, 1 out]
        n391 = call "Select_Table_Vaule Enable_Disable.vi"("Action"=w997, "Table"=w996) -> ("Enable"=w995:bool)  [unwired: 8 in, 1 out]
        n392 = case shown="True" w995 {
          tunnel: w1003 -> [w1019 w1042]
          tunnel: [w1019 w1041] -> w983
          tunnel: [w1016 w1034] -> w998
          tunnel: w997 -> [_ w1038]
          tunnel: w996 -> [_ w1043]
          tunnel: w994 -> [_ _]
          tunnel: [w1017 w1032] -> w967
          tunnel: [_ w1040] -> w992
          tunnel: [_ w1033] -> w985
          tunnel: T7[] ["eol_bemf_mp_cold_coef_a", "eol_bemf_mp_cold_coef_b", "eol_bemf_mp_cold_coef_c", "eol_bemf_lsi_cold_ref_coeffs", "eol_bemf_lsi_speed", "eol_bemf_lsi_integral_0", "eol_bemf_lsi_integral_1", "eol_bemf_lsi_integral_2", "eol_cold_bemf", "eol_cold_bemf_fisf"] ("Calibration") -> [_ w1030]
          tunnel: [w1014 w1024] -> w984
          tunnel: [w1014 w1020] -> w956
          frame False {
            w1016 = "Skip" ("software string")
            n393 = Initialize Array(w1016, 10 ("维数大小")) -> (w1014:string[])
            n394 = Build Array(TRUE) -> (w1017:bool[])
          }
          frame True {
            n395 = for {
              tunnel: [w1044] -> w1040 mode=indexing
              tunnel: [w1048] -> w1033
              tunnel: w1030 -> [w1047] mode=indexing
              tunnel: [w1046] -> w1029 mode=indexing
              shift-right: [w1050] -> w1041
              shift-left: w1042 -> [w1051]
              n396 = Build Array(w1047) -> (w1045:T7[])
              n397 = call "get_calibration.vi"("Calibration"=w1045, "daemon reference in"=w1051) -> ("error out"=w1048:errorcluster, "response"=w1046:string, "values"=w1049:dbl[], "daemon reference out"=w1050:refnum<k5>)  [unwired: 5 in, 1 out]
              n398 = Index Array(array=w1049) -> (element=w1044:dbl)  [unwired: 1 in]
            }
            n399 = Number To Fractional String(number=w1040) -> (F-format string=w1024:string[])  [unwired: 3 in]
            n400 = Build Array (concatenate)(w1038, string[] ["Read_eol_bemf_mp_cold_coef_a_A", "Read_eol_bemf_mp_cold_coef_b_A", "Read_eol_bemf_mp_cold_coef_c_A", "Read_eol_bemf_lsi_cold_ref_coeffs_A", "Read_eol_bemf_lsi_speed_A", "Read_eol_bemf_lsi_integral_0_A", "Read_eol_bemf_lsi_integral_1_A", "Read_eol_bemf_lsi_integral_2_A", "Read_eol_cold_bemf_A", "Read_eol_cold_bemf_fisf_A"]) -> (w1039:string[])
            n401 = Interleave 1D Arrays(w1030, w1024) -> (w1037:T7[])
            n402 = Array To Spreadsheet String(delimiter (Tab)=",", array=w1029, 3:"" ("format string")) -> (spreadsheet string=w1028:string)
            n403 = Array To Spreadsheet String(delimiter (Tab)=";" ("分隔符(Tab)"), array=w1037, 3:"" ("格式字符串")) -> (spreadsheet string=w1034:string)
            n404 = Build Array (concatenate)(w1028, w1024) -> (w1031:string[])
            n405 = for {
              tunnel: w1039 -> [w1058] mode=indexing
              tunnel: w1043 -> [w1057]
              tunnel: w1031 -> [w1055] mode=indexing
              tunnel: [w1054] -> w1032 mode=indexing
              tunnel: [w1052] -> w1021 mode=indexing
              w1063 = "UIdisplay" ("Process (\"\" - local)")
              n406 = call <vilib>:"Trim Whitespace.vi"("string"=w1058) -> ("trimmed string"=w1053:string)  [unwired: 1 in]
              n407 = call "Select_Table_Vaule.vi"("Vaule"=w1055, "Action"=w1053, "Table"=w1057) -> ("Result"=w1054:bool, "vaule"=w1056:string[])  [unwired: 7 in]
              n408 = Append True/False String(1:w1054, 2:"FAIL" ("真字符串"), 3:"PASS" ("真字符串")) -> (0:w1052:string)  [unwired: 1 in]
              n409 = Build Array (concatenate)(w1056, w1055, w1052) -> (w1062:string[])
              n410 = Flatten To XML(anything=w1062) -> (xml string=w1061:string)
              n411 = call "AMC Send Local Message.vi"("Process (\"\" - local)"=w1063, "Message Value"=w1061, "Message Name"=w1063) -> ()  [unwired: 7 in, 2 out]
            }
            n412 = Delete From Array(array=w1021, length=1 ("长度"), index=0 ("索引")) -> (array with subset deleted=w1020:string[])  [unwired: 1 out]
          }
        }
        n413 = property class="Bool (严格)"(reference=w977) -> ("Value"=w979:bool)  [unwired: 1 in, 2 out]
        n414 = Unbundle By Name(w976) -> ("Fail_resume_mode"=w978:bool)
        n415 = Not(x=w979) -> (.not. x?=w980:bool)
        n416 = Or(x=w978, y=w980) -> (x .or. y?=w971:bool)
        n417 = call <vilib>:"Space Constant.vi"() -> ("String"=w1000:string)
        n418 = Concatenate Strings(w997, w1000, w998) -> (w999:string)
        n419 = Index Array(array=w956) -> (element #1=w955:string, element #2=w954:string, element #3=w953:string, element #4=w952:string, element #5=w951:string, element #6=w950:string, element #7=w949:string, element #8=w948:string, element #9=w947:string, element #10=w946:string)  [unwired: 10 in]
        n420 = Index Array(array=w984) -> (element #1=w966:string, element #2=w965:string, element #3=w964:string, element #4=w963:string, element #5=w962:string, element #6=w961:string, element #7=w960:string, element #8=w959:string, element #9=w958:string, element #10=w957:string)  [unwired: 10 in]
        n421 = Delete From Array(array=w967, length=1 ("长度"), index=0 ("索引")) -> (array with subset deleted=w988:bool[])  [unwired: 1 out]
        n422 = Select(t="Calibration_Read_and_check_Calibration_value_B", s=w971, f="Calibration_Save_Calibration") -> (s? t:f=w968:string)
        n423 = And Array Elements(Boolean array=w988) -> (logical AND=w973:bool)
        n424 = Bundle By Name(cluster=w986, "daemon reference"=w983, "BEMF_Calibration.Calibration Result - eol_bemf_mp_cold_coef_a"=w966, "BEMF_Calibration.Calibration Result - eol_bemf_mp_cold_coef_b"=w965, "BEMF_Calibration.Calibration Result - eol_bemf_mp_cold_coef_c"=w964, "BEMF_Calibration.Calibration Result - eol_bemf_lsi_cold_ref_coeffs"=w963, "BEMF_Calibration.Get - Calibration Result - eol_bemf_lsi_speed"=w962, "BEMF_Calibration.Get - Calibration Result - eol_bemf_lsi_integral_0"=w961, "BEMF_Calibration.Calibration Result - eol_bemf_lsi_integral_1"=w960, "BEMF_Calibration.Get - Calibration Result - eol_bemf_lsi_integral_2"=w959, "BEMF_Calibration.Get - Calibration Result - eol_cold_bemf"=w958, "BEMF_Calibration.Get - Calibration Result - eol_cold_bemf_fisf"=w957, "BEMF_Calibration_Status.Calibration Result - eol_bemf_mp_cold_coef_a"=w955, "BEMF_Calibration_Status.Calibration Result - eol_bemf_mp_cold_coef_b"=w954, "BEMF_Calibration_Status.Calibration Result - eol_bemf_mp_cold_coef_c"=w953, "BEMF_Calibration_Status.Calibration Result - eol_bemf_lsi_cold_ref_coeffs"=w952, "BEMF_Calibration_Status.Get - Calibration Result - eol_bemf_lsi_speed"=w951, "BEMF_Calibration_Status.Get - Calibration Result - eol_bemf_lsi_integral_0"=w950, "BEMF_Calibration_Status.Calibration Result - eol_bemf_lsi_integral_1"=w949, "BEMF_Calibration_Status.Get - Calibration Result - eol_bemf_lsi_integral_2"=w948, "BEMF_Calibration_Status.Get - Calibration Result - eol_cold_bemf"=w947, "BEMF_Calibration_Status.Get - Calibration Result - eol_cold_bemf_fisf"=w946) -> (w982:T2)
        n425 = Bundle By Name(cluster=w1002, "BEMF_Calibration.Calibration_Vaule"=w992, "BEMF_Calibration.Calibration_Vaule_status"=w988) -> (w1001:T3)
        n426 = Select(t=TRUE, s=w971, f=w973) -> (s? t:f=w972:bool)
        n427 = case shown="No Error" w985 {
          tunnel: [w1010 "Error"] -> w993
          tunnel: w972 -> [w1009 _]
          tunnel: [w1008 TRUE] -> w987
          tunnel: w968 -> [_ _]
          frame No Error {
            n428 = Not(x=w1009) -> (.not. x?=w1008:bool)
            n429 = Select(t="Calibration_Save_Calibration", s=w1009, f="Finalization_NG_unit") -> (s? t:f=w1010:string)
          }
          frame Error {
          }
        }
        n430 = call "LogStatus.vi"("error in (no error)"=w985, "last message"=w1004, "message"=w999) -> ("error  out"=w1005:errorcluster)  [unwired: 8 in]
      }
      frame "Calibration_Save_Calibration" {
        n431 = Unbundle By Name(w1065) -> ("MES bool"=w1068:refnum<vi>)
        n432 = call "HD_Config.vi"("Step"=enum16{"Initial", "Write", "Read"}."Read") -> ("HD Config out"=w1067:T5)  [unwired: 9 in, 1 out]
        n433 = property class="Bool (严格)"(reference=w1068) -> ("Value"=w1070:bool)  [unwired: 1 in, 2 out]
        n434 = Unbundle By Name(w1067) -> ("Fail_resume_mode"=w1069:bool)
        n435 = Unbundle By Name(w1077) -> ("Table"=w1084:string[][], "daemon reference"=w1089:refnum<k5>, "Config"=w1082:string[][])
        n436 = Not(x=w1070) -> (.not. x?=w1071:bool)
        n437 = Or(x=w1069, y=w1071) -> (x .or. y?=w1064:bool)
        n438 = call "Select_Table_Vaule Enable_Disable.vi"("Action"=w1085, "Table"=w1084) -> ("Enable"=w1083:bool)  [unwired: 8 in, 1 out]
        n439 = case shown="True" w1083 {
          tunnel: w1089 -> [w1096 w1106]
          tunnel: [w1096 w1105] -> w1075
          tunnel: [w1095 w1097] -> w1079
          tunnel: w1085 -> [_ w1104]
          tunnel: w1084 -> [_ w1103]
          tunnel: w1082 -> [_ _]
          tunnel: [_ w1100] -> w1076
          tunnel: [w1095 w1097] -> w1073
          tunnel: [w1095 w1099] -> w1072
          tunnel: w1064 -> [_ w1098]
          frame False {
            w1095 = "Skip" ("software string")
            (unwired) TRUE
          }
          frame True {
            w1109 = "UIdisplay" ("Process (\"\" - local)")
            n440 = case shown="False" w1098 {
              tunnel: w1106 -> [w1119 w1121]
              tunnel: [w1118 w1121] -> w1105
              tunnel: [w1117 _] -> w1100
              tunnel: [w1116 "Skip" ("response")] -> w1097
              frame False {
                n441 = call "finalise_calibration.vi"("daemon reference in"=w1119) -> ("error out"=w1117:errorcluster, "response"=w1116:string, "daemon reference out"=w1118:refnum<k5>)  [unwired: 7 in, 1 out]
                n442 = call "Time Delay"("error in (no error)"=w1117, "Delay Time (s)"=1.0) -> ()  [unwired: 9 in, 1 out]
              }
              frame True {
              }
            }
            n443 = call "Select_Table_Vaule.vi"("Vaule"=w1097, "Action"=w1104, "Table"=w1103) -> ("Result"=w1101:bool, "vaule"=w1102:string[])  [unwired: 7 in]
            n444 = case shown="False" w1098 {
              tunnel: w1101 -> [w1111 _]
              tunnel: [w1110 "Skip" ("response")] -> w1099
              frame False {
                n445 = Append True/False String(1:w1111, 2:"FAIL" ("真字符串"), 3:"PASS" ("真字符串")) -> (0:w1110:string)  [unwired: 1 in]
              }
              frame True {
              }
            }
            n446 = Build Array (concatenate)(w1102, w1097, w1099) -> (w1108:string[])
            n447 = Flatten To XML(anything=w1108) -> (xml string=w1107:string)
            n448 = call "AMC Send Local Message.vi"("Process (\"\" - local)"=w1109, "Message Value"=w1107, "Message Name"=w1109) -> ()  [unwired: 7 in, 2 out]
          }
        }
        n449 = call <vilib>:"Space Constant.vi"() -> ("String"=w1088:string)
        n450 = Concatenate Strings(w1085, w1088, w1079) -> (w1087:string)
        n451 = Bundle By Name(cluster=w1077, "daemon reference"=w1075, "BEMF_Calibration.Finalise Calibration"=w1073, "BEMF_Calibration_Status.Finalise Calibration"=w1072) -> (w1074:T2)
        n452 = call "LogStatus.vi"("error in (no error)"=w1076, "last message"=w1090, "message"=w1087) -> ("error  out"=w1091:errorcluster)  [unwired: 8 in]
        n453 = case shown="Error" w1076 {
          tunnel: [_ TRUE] -> w1080
          tunnel: [_ "Error"] -> w1081
          frame No Error {
          }
          frame Error {
          }
        }
      }
      frame "Calibration_Read_and_check_Calibration_value_B" {
        n454 = Unbundle By Name(w1131) -> ("Table"=w1144:string[][], "daemon reference"=w1143:refnum<k5>)
        n455 = Unbundle By Name(w1156) -> ("BEMF_Calibration.Calibration_Vaule"=w1145:dbl[])
        n456 = call "Select_Table_Vaule Enable_Disable.vi"("Action"=w1151, "Table"=w1144) -> ("Enable"=w1150:bool)  [unwired: 8 in, 1 out]
        n457 = case shown="False" w1150 {
          tunnel: w1143 -> [w1168 w1195]
          tunnel: [w1168 w1194] -> w1126
          tunnel: [w1167 w1187] -> w1152
          tunnel: w1151 -> [_ w1192]
          tunnel: w1144 -> [_ w1196]
          tunnel: [_ w1177] -> w1147
          tunnel: [_ w1186] -> w1129
          tunnel: T7[] ["eol_cold_bemf", "eol_cold_bemf_fisf"] ("Calibration") -> [_ w1185]
          tunnel: w1145 -> [_ w1180]
          tunnel: [_ w1175] -> w1128
          tunnel: [w1166 w1172] -> w1127
          tunnel: [_ w1170] -> _
          tunnel: [_ w1169] -> _
          frame False {
            w1167 = "Skip" ("software string")
            n458 = Initialize Array(w1167, 3 ("维数大小")) -> (w1166:string[])
          }
          frame True {
            n459 = for {
              tunnel: [w1197] -> w1177 mode=indexing
              tunnel: [w1201] -> w1186
              tunnel: w1185 -> [w1200] mode=indexing
              tunnel: [w1199] -> w1184 mode=indexing
              shift-right: [w1203] -> w1194
              shift-left: w1195 -> [w1204]
              n460 = Build Array(w1200) -> (w1198:T7[])
              n461 = call "get_calibration.vi"("Calibration"=w1198, "daemon reference in"=w1204) -> ("error out"=w1201:errorcluster, "response"=w1199:string, "values"=w1202:dbl[], "daemon reference out"=w1203:refnum<k5>)  [unwired: 5 in, 1 out]
              n462 = Index Array(array=w1202) -> (element=w1197:dbl)  [unwired: 1 in]
            }
            n463 = Array Subset(array=w1180, index=8, length=2) -> (w1176:dbl[])
            n464 = Number To Fractional String(number=w1177) -> (F-format string=w1191:string[])  [unwired: 3 in]
            n465 = Build Array (concatenate)(w1192, string[] ["Read_eol_cold_bemf_B", "Read_eol_cold_bemf_fisf_B"]) -> (w1193:string[])
            n466 = Interleave 1D Arrays(w1185, w1191) -> (w1190:T7[])
            n467 = Array To Spreadsheet String(delimiter (Tab)=";", array=w1184, 3:"" ("format string")) -> (spreadsheet string=w1171:string)
            n468 = Array To Spreadsheet String(delimiter (Tab)=";" ("分隔符(Tab)"), array=w1190, 3:"" ("格式字符串")) -> (spreadsheet string=w1187:string)
            n469 = Build Array (concatenate)(w1171, w1191) -> (w1170:string[])
            n470 = Equal?(x=w1177, y=w1176) -> (x = y?=w1175:bool[])
            n471 = Build Array (concatenate)(TRUE, w1175) -> (w1173:bool[])
            n472 = for {
              tunnel: w1193 -> [w1217] mode=indexing
              tunnel: w1196 -> [w1216]
              tunnel: w1170 -> [w1214] mode=indexing
              tunnel: w1173 -> [w1211]
              tunnel: [w1209] -> w1172 mode=indexing
              tunnel: [w1205] -> w1169 mode=indexing
              i -> [w1210]
              w1220 = "UIdisplay" ("Process (\"\" - local)")
              n473 = call <vilib>:"Trim Whitespace.vi"("string"=w1217) -> ("trimmed string"=w1213:string)  [unwired: 1 in]
              n474 = Equal To 0?(x=w1210) -> (x = 0?=w1212:bool)
              n475 = call "Select_Table_Vaule.vi"("Vaule"=w1214, "Action"=w1213, "Table"=w1216) -> ("Result"=w1206:bool, "vaule"=w1215:string[])  [unwired: 7 in]
              n476 = case shown="False" w1212 {
                tunnel: w1206 -> [_ w1228]
                tunnel: [w1224 w1227] -> w1209
                tunnel: w1211 -> [w1223 _]
                tunnel: w1210 -> [w1221 _]
                frame False {
                  n477 = Index Array(array=w1223, index=w1221) -> (element=w1222:bool)
                  n478 = Append True/False String(1:w1222, 2:"FAIL" ("真字符串"), 3:"PASS" ("真字符串")) -> (0:w1224:string)  [unwired: 1 in]
                }
                frame True {
                  n479 = Append True/False String(1:w1228, 2:"FAIL" ("真字符串"), 3:"PASS" ("真字符串")) -> (0:w1227:string)  [unwired: 1 in]
                }
              }
              n480 = Build Array (concatenate)(w1215, w1214, w1209) -> (w1219:string[])
              n481 = Flatten To XML(anything=w1219) -> (xml string=w1218:string)
              n482 = Append True/False String(1:w1206, 2:"FAIL" ("真字符串"), 3:"PASS" ("真字符串")) -> (0:w1205:string)  [unwired: 1 in]
              n483 = call "AMC Send Local Message.vi"("Process (\"\" - local)"=w1220, "Message Value"=w1218, "Message Name"=w1220) -> ()  [unwired: 7 in, 2 out]
            }
          }
        }
        n484 = call <vilib>:"Space Constant.vi"() -> ("String"=w1154:string)
        n485 = Concatenate Strings(w1151, w1154, w1152) -> (w1153:string)
        n486 = Unbundle By Name(w1132) -> ("MES bool"=w1138:refnum<vi>)
        n487 = call "HD_Config.vi"("Step"=enum16{"Initial", "Write", "Read"}."Read") -> ("HD Config out"=w1137:T5)  [unwired: 9 in, 1 out]
        n488 = property class="Bool (严格)"(reference=w1138) -> ("Value"=w1140:bool)  [unwired: 1 in, 2 out]
        n489 = Unbundle By Name(w1137) -> ("Fail_resume_mode"=w1139:bool)
        n490 = Not(x=w1140) -> (.not. x?=w1141:bool)
        n491 = Or(x=w1139, y=w1141) -> (x .or. y?=w1142:bool)
        n492 = And Array Elements(Boolean array=w1128) -> (logical AND=w1133:bool)
        n493 = Select(t=TRUE, s=w1142, f=w1133) -> (s? t:f=w1134:bool)
        n494 = Index Array(array=w1127, index #1=1 ("索引"), index #2=2 ("索引")) -> (element #1=w1123:string, element #2=w1122:string)
        n495 = case shown="Error" w1129 {
          tunnel: [w1161 "Error"] -> w1149
          tunnel: w1134 -> [w1160 _]
          frame No Error {
            n496 = Select(t="Power_Tunings_and_AW_Performance_Test", s=w1160, f="Finalization_NG_unit") -> (s? t:f=w1161:string)
          }
          frame Error {
          }
        }
        n497 = Bundle By Name(cluster=w1131, "daemon reference"=w1126, "BEMF_Calibration.Compare -Calibration Result - eol_cold_bemf"=w1123, "BEMF_Calibration.Compare -Calibration Result - eol_cold_bemf_fisf"=w1122, "BEMF_Calibration_Status.Compare -Calibration Result - eol_cold_bemf"=w1123, "BEMF_Calibration_Status.Compare -Calibration Result - eol_cold_bemf_fisf"=w1122) -> (w1130:T2)
        n498 = Bundle By Name(cluster=w1156, "BEMF_Calibration.Calibration_Vaule _B"=w1147, "BEMF_Calibration.Calibration_Vaule_B_status"=w1128) -> (w1155:T3)
        n499 = call "LogStatus.vi"("error in (no error)"=w1129, "last message"=w1157, "message"=w1153) -> ("error  out"=w1158:errorcluster)  [unwired: 8 in]
      }
    }
    n500 = call "Stop.vi"("Step"=enum16{"Initial", "Write", "Read"}."Read") -> ("Stop Out"=w26:bool)  [unwired: 9 in, 1 out]
    n501 = call "Exit.vi"("Step"=enum16{"Initial", "Write", "Read"}."Read" ("step")) -> ("Exit Out"=w25:bool)  [unwired: 9 in, 1 out]
    n502 = call "6-AlarmStatus.vi"("Step"=enum16{"Initial", "Write", "Read"}."Read") -> ("AlarmValue Out"=w18:bool[])  [unwired: 9 in, 1 out]
    n503 = Or Array Elements(Boolean array=w18) -> (logical OR=w17:bool)
    n504 = Compound Arithmetic op=OR(w24, w26, w25, w17) -> (w23:bool)
    n505 = call "AMC Run Step.vi"("Message Queue In"=w44, "Message Name"=w32, "Message Value"=w30, "error in (no error)"=w39, "Mli/Sig"=FALSE) -> ("Message Queue Out"=w43:T4, "error out"=w38:errorcluster)  [unwired: 13 in]
  }
  "Message Queue Out" <- w5
  "error out" <- w4
  "Data" <- w10
  "Flow" <- w7
  "Data out" <- w2
